vi "Text control 2 v3.6.vi"() -> ()   [LabVIEW 2016]
panel:
  in  "Delay before read (ms)":u32=1000
  out "I vs Vd":cluster{"Y data in":dbl[], "X data in":dbl[]}[](graph)
  in  "Auto Reset":bool
  in  "Reset":bool
  out "Id min vs time":cluster{"Y data in":dbl[], "X data in":dbl[]}[](graph)
  in  "Time Offset":dbl caption="Set Start Time (s)"
  out "Total lines":i32
  out "Line running":i32
  in  "byte count":u32=64
  in  "Serial End Mode for Reads":u16(ring)=2 items=["None", "LastBit", "TermChar"]
  in  "Timeout (ms)":u32=10000
  in  "Enable Termination\nChar (T)":bool=TRUE
  in  "Termination char\n(0xA = '\\n' = LF)\n(0xD = '\\r' = CR)":u8=13 format="%.0x"
  in  "flow control":u16(ring) items=["None"=0, "XON/XOFF"=1, "RTS/CTS"=2, "DTR/DSR"=4]
  in  "stop bits":u16(ring)=10 items=["1.0"=10, "1.5"=15, "2.0"=20]
  in  "parity":u16(ring) items=["None", "Odd", "Even", "Mark", "Space"]
  in  "data bits":u16=8 min=5 max=8 step=1
  in  "VISA resource name":refnum<visa-resource-name>="COM6"
  in  "baud rate":u32=9600
  out "Serial port output":string
  out "error out":errorcluster
  in  "Units":u16(ring) items=["Seconds", "Minutes", "Hours"]
  out "Elapsed Time":dbl caption="Elapsed Time (s)"
  out "Id max vs time":cluster{"Y data in":dbl[], "X data in":dbl[]}[](graph)
  out "Ig":dbl format="%.2e"
  out "Id":dbl format="%.2e"
  out "Is":dbl format="%.2e"
  out "I vs Vg":cluster{"Y data in":dbl[], "X data in":dbl[]}[](graph)
  in  "Panel Controls 2":T1={"Emergency Stop"=refnum, "TransGraph Max"=1e-05, "Text/Graph (text=false)"=TRUE, "TransGraph Min"=1e-11} {"TransGraph Min" format="%.2e"; "TransGraph Max" format="%.2e"}
  out "Command running:":string="#output s 0 0 0 -0.008 0.008 0.002"
  in  "Standby":T2
  in  "Full Reset":bool
  in  "SMU4":cluster{"on/off":bool, "Voltage":dbl} {"Voltage" min=-100.0 max=100.0 format="%.2f"}
  in  "Source/Drain Range":u8(slide)=6 max=11 scale=0.0..11.0
  in  "Source/Drain\nRange mode":u16(ring) items=["Auto", "Limited", "Fixed"]
  in  "Gate Range":u8(slide)=6 max=11 scale=0.0..11.0
  in  "Gate Range\nmode":u16(ring) items=["Auto", "Limited", "Fixed"]
  in  "Gate":T3={"Gate Start"=0.0, "Gate Stop"=2.0, "Gate Step (linear only)"=1.0, "Gate Compliance"=0.0001, "Gate PComp"=0.0, "Range mode"=0, "Range"=6} {"Range" max=11 scale=0.0..11.0; "Range mode" items=["Auto", "Limited", "Fixed"]; "Gate PComp" format="%^.2e"; "Gate Compliance" format="%^.2e"; "Gate Step (linear only)" format="%^.4e"; "Gate Stop" format="%^.4e"; "Gate Start" format="%^.4e"}
  in  "Drain 2":T4={"Drain Start"=0.0, "Drain Stop"=2.0, "Drain Compliance"=0.0001, "Drain Step"=1.0, "Drain PComp"=0.0, "Range mode"=0, "Range"=6} {"Range" max=11 scale=0.0..11.0; "Range mode" items=["Auto", "Limited", "Fixed"]; "Drain PComp" format="%^.2e"; "Drain Step" format="%^.4e"; "Drain Compliance" format="%^.2e"; "Drain Stop" format="%^.4e"; "Drain Start" format="%^.4e"}
  in  "Timings 2":T5={"integration time"=0, "Short/Long integration time"=0.00064, "hold time (sec)"=0.0, "delay time (sec)"=0.0, "Step Time (0 disables)"=0.0, "sweep method"=0, "Pulse period"=0.005, "Base voltage"=0.0, "Pulse width"=0.0005} {"Pulse width" min=0.0005 max=0.1 step=0.0001 format="%.4f"; "Base voltage" format="%^.4e"; "Pulse period" min=0.005 max=1.0 step=0.0001 format="%.4f"; "sweep method" items=["Continuous", "Pulsed"]; "Step Time (0 disables)" format="%.2f"; "delay time (sec)" format="%.4f"; "hold time (sec)" format="%.4f"; "Short/Long integration time" format="%^.0e"; "integration time" scale=0.0..2.0}
  in  "Panel Controls":T6={"Emergency Stop"=refnum, "TransGraph Max"=1e-05, "Text/Graph (text=false)"=TRUE} {"TransGraph Max" format="%.2e"}
  in  "Interrupt run":bool
  in  "Drain: Compliance":dbl=0.001 format="%.8f"
  in  "Gate: Compliance":dbl=0.001 format="%.8f"
  out "Path":path=path "C:/users/rlp38/09Apr2009LTtesting/test2.txt"
  in  "hold time /s":dbl format="%.2f"
  in  "delay time /s":dbl format="%.2f"
  in  "integration time":u32(slide) max=2 step=1 scale=0.0..2.0
  in  "Integration time (short)":dbl=0.0019 min=8e-05 max=0.0019 step=8e-05 format="%^.0e"
  in  "Integration time (long)":dbl=0.32 min=0.04 max=2.0 step=0.02 format="%.2f"
  in  "Step delay /s":dbl format="%.2f"
  in  "Program":string="#pulsedstressV d 0.03 20 0 0.5 0.0827 5\n#\n#itime s\n#gaterangemode l\n#drainrangemode l\n#serial /1Q\n#serial /1ZR\n#pulsed on 0.05 0 0.02\n#transfer d 1 -1 -0.1 -1 -1 0\n#wait-min 1\n#transfer d 1 -1 -0.1 -1 -1 0\n#output d 0 -1 -0.5 0 -1 -0.1\n#transfer d -10 40 1 5 40 35\n#transfer d -10 40 1 5 40 35\n#output d 0 40 20 0 40 1\n#\n#\n#sample 1 0.008 221 6 0.003\n#samplei 400e-6 200 6 0.002 0.1\n#vsu2pulse -10 4\n#\n#stressV 0.016 0.03 2e-4 0.1e-3 11\n#stressI 220e-7 0.08 15\n#transfer s -1 1 0.5 -0.005 0.005 0.005\n#output s 0 0 0 -0.008 0.008 0.002"
  # "Serial port settings"
  # "Time"
  # "Syntax:\nitime [s|m|l]\ngaterangemode [a|l|f]\ndrainrangemode [a|l|f]\npulsed [on|off] PulsePeriod(sec) PulseBaseVoltage PulseONWidth(sec)\nstandby [on l off]\nwait NumMilliseconds\nwait-min NumMinutes\n# texthere = comment\ntransfer [s|d] VgStart VgStop VgStep VdStart VdStop VdStep\noutput [s|d] VgStart VgStop VgStep VdStart VdStop VdStep\nsample Vg Vd NumSamples Time(s) SampleInterval(s)\nsamplei Idg NumSamples Time(s) SampleInterval(s) VDGcompliance\n100 samples is approximately 13 seconds with medium integration\n# if in doubt use SampleInterval(s) = 0.004\nstressV VG VD IGcompliance IDcompliance Duration(sec)\nstressI IDG VDGcompliance Duration(sec)\nvsu2pulse Bias Duration(s)\npulsedstressV [s|d] VEstop VgON VgOFF Period(s) PulseONwidth(s) Vd\nsample-fpp Vg Vd NumSamples Time\nresample-fpp Vg Vd\ntransfer-fpp [s|d] VgStart VgStop VgStep VdStart VdStop VdStep\noutput-fpp [s|d] VgStart VgStop VgStep VdStart VdStop VdStep\nserial SerialPortCommand\n\nSPM OEM Pump Syntax (x: pump number, use 1 if only one pump):\n/xQ: query\n/xZR: initialize pump\n/xIn: turn to port number n (clockwise)\n/xOn: turn to port number n (counterclockwise)"
  # "1\n2\n3\n4\n5\n6\n7\n8\n9\n10\n11\n12\n13\n14\n15\n16\n17\n18\n19\n20\n21\n22\n23\n24\n25"
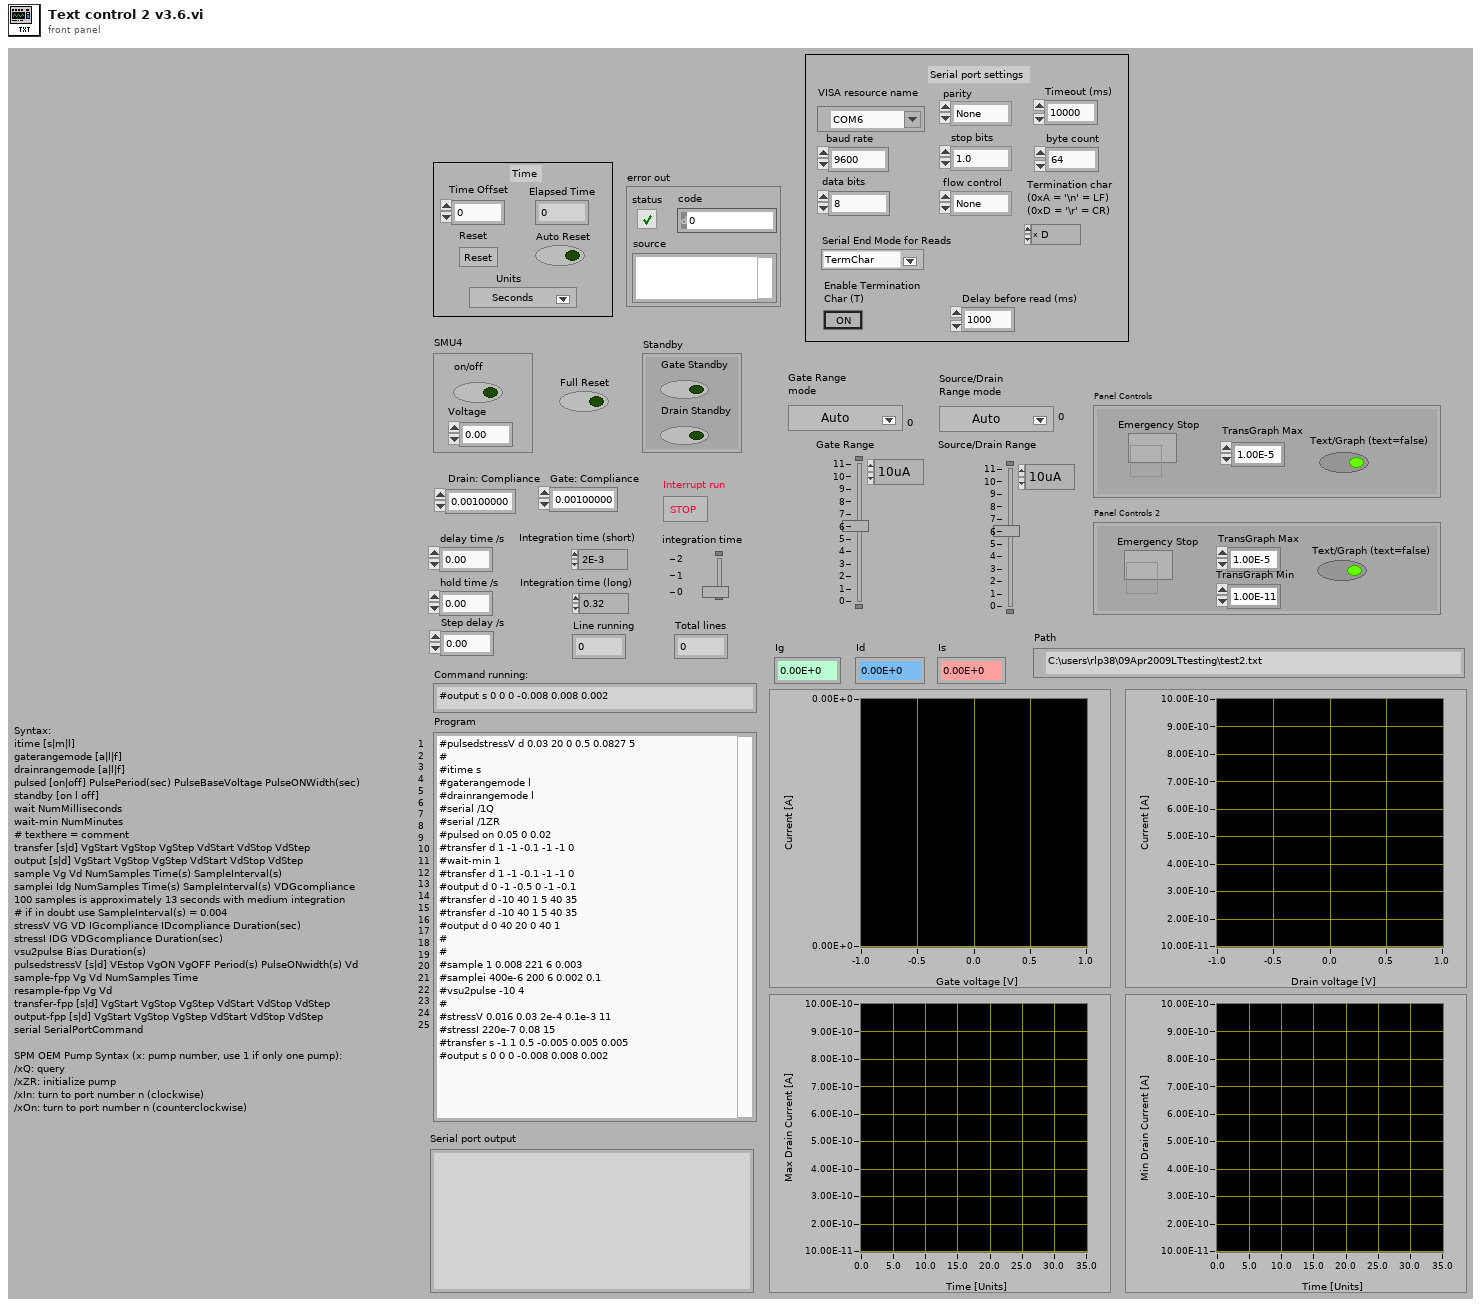
[diagram p1: front panel]
types:
  T1 = cluster{"Emergency Stop":refnum<vi>, "TransGraph Max":dbl, "Text/Graph (text=false)":bool, "TransGraph Min":dbl}
  T2 = cluster{"Gate Standby":bool, "Drain Standby":bool}
  T3 = cluster{"Gate Start":dbl, "Gate Stop":dbl, "Gate Step (linear only)":dbl, "Gate Compliance":dbl, "Gate PComp":dbl, "Range mode":u16, "Range":u8}
  T4 = cluster{"Drain Start":dbl, "Drain Stop":dbl, "Drain Compliance":dbl, "Drain Step":dbl, "Drain PComp":dbl, "Range mode":u16, "Range":u8}
  T5 = cluster{"integration time":u32, "Short/Long integration time":dbl, "hold time (sec)":dbl, "delay time (sec)":dbl, "Step Time (0 disables)":dbl, "sweep method":u16, "Pulse period":dbl, "Base voltage":dbl, "Pulse width":dbl}
  T6 = cluster{"Emergency Stop":refnum<vi>, "TransGraph Max":dbl, "Text/Graph (text=false)":bool}
  T7 = enum16{"open", "replace", "create", "open or create", "replace or create", "replace or create with confirmation"}
  T8 = cluster{"V2 Start":dbl, "V2 Step":dbl, "Number of points":i32}
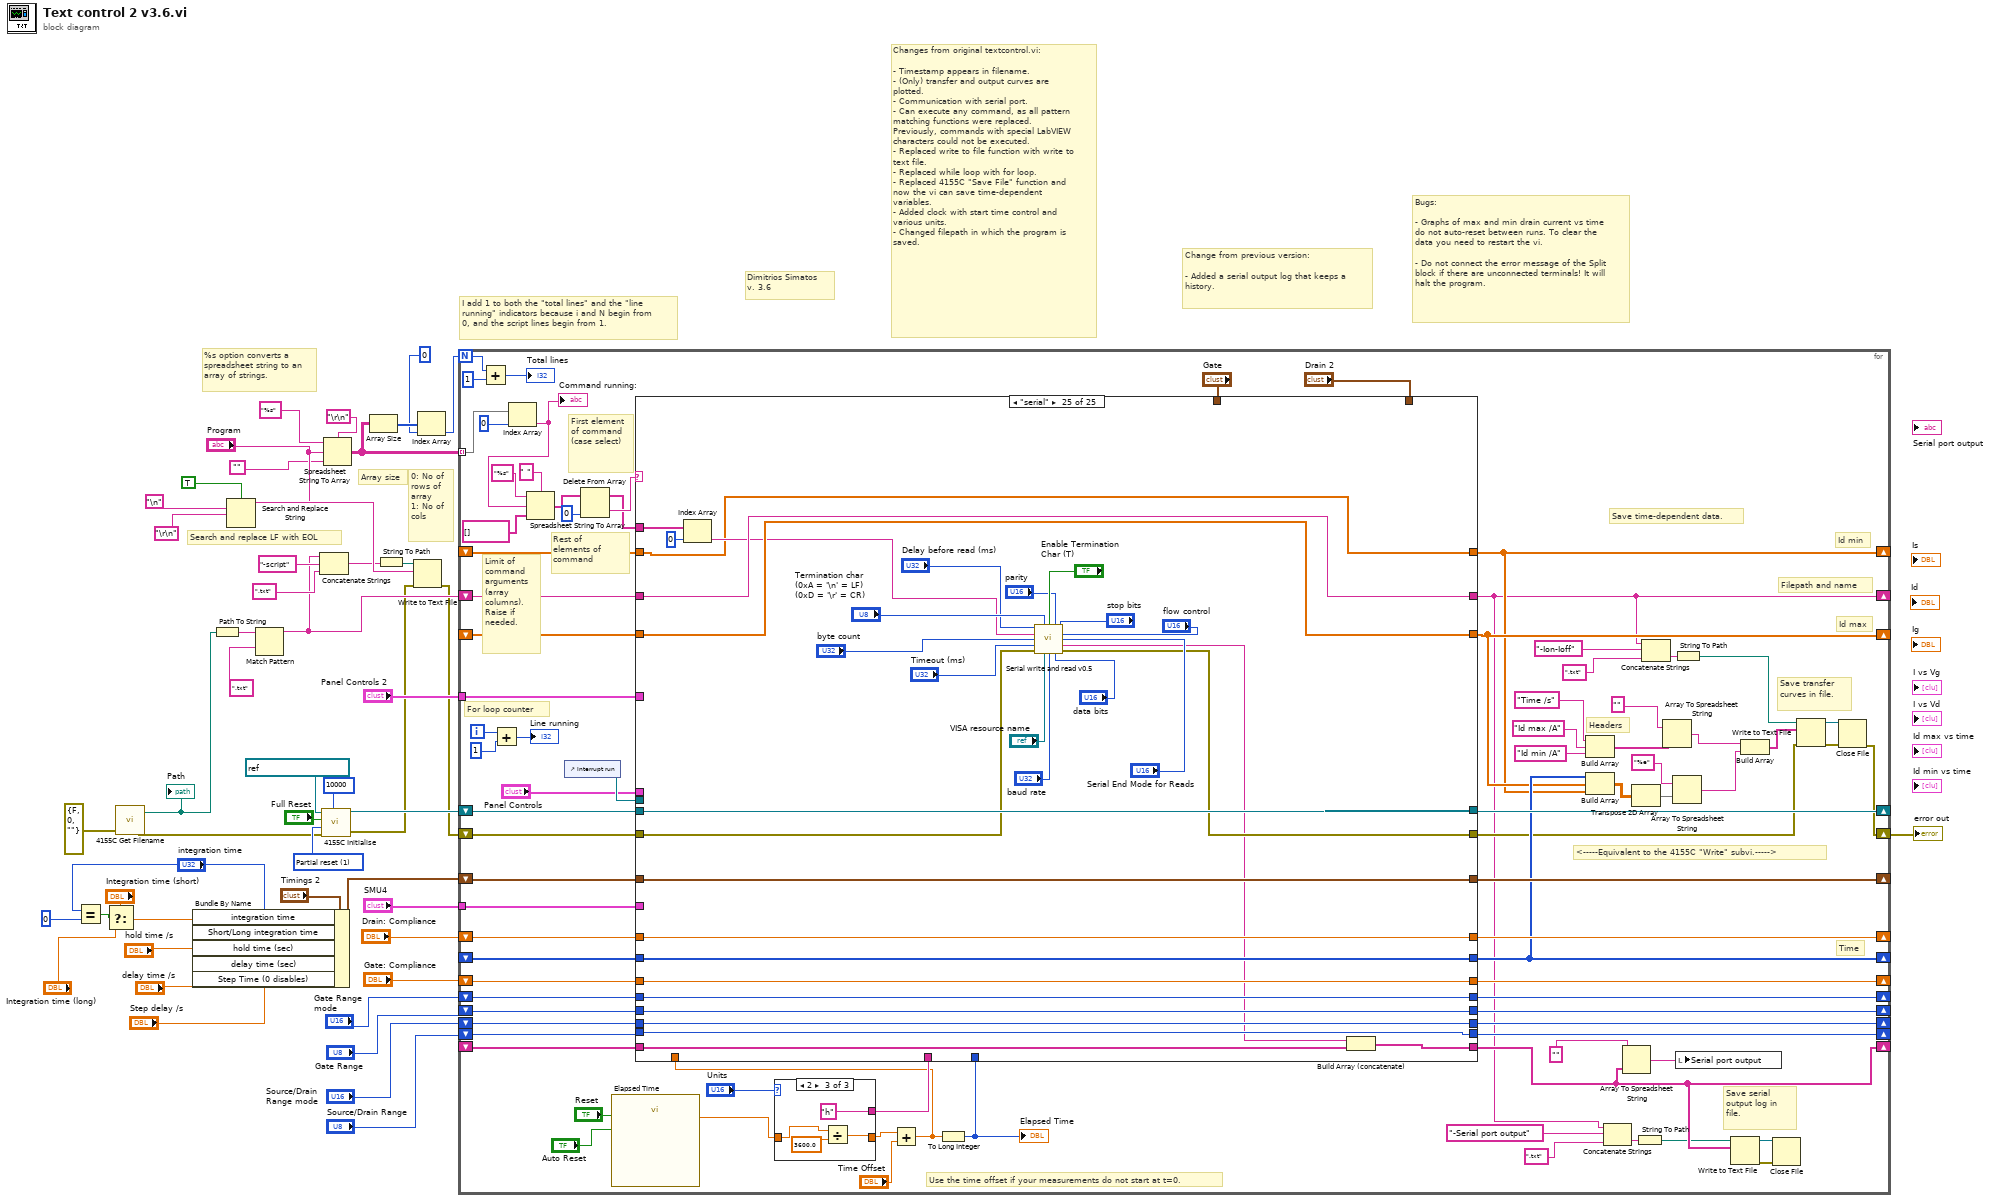
[diagram p0: block diagram]
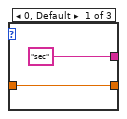
[diagram p2: hidden frame]
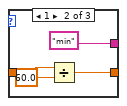
[diagram p3: hidden frame]
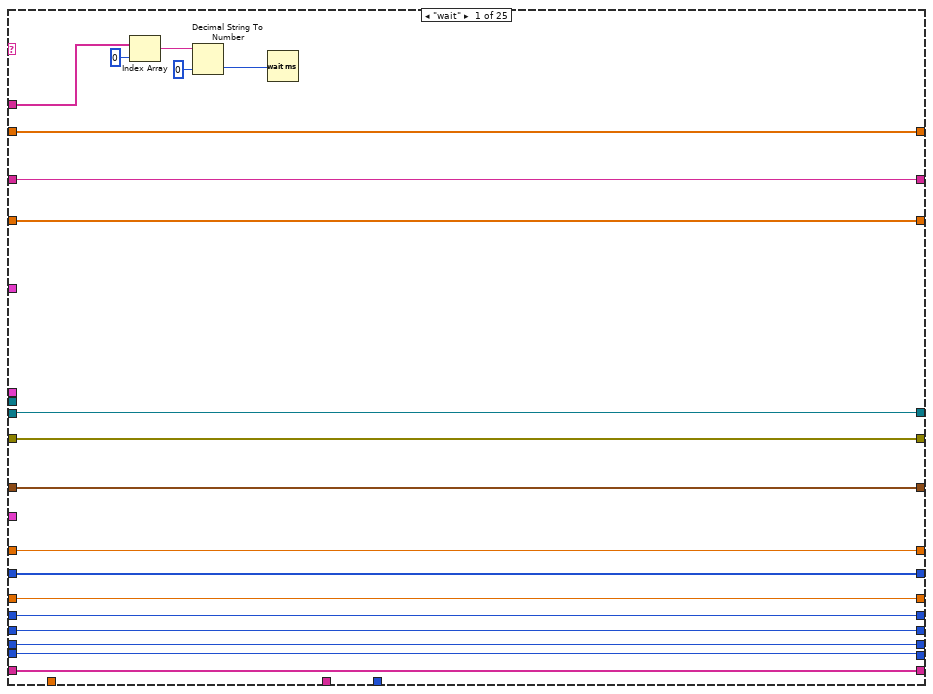
[diagram p4: hidden frame]
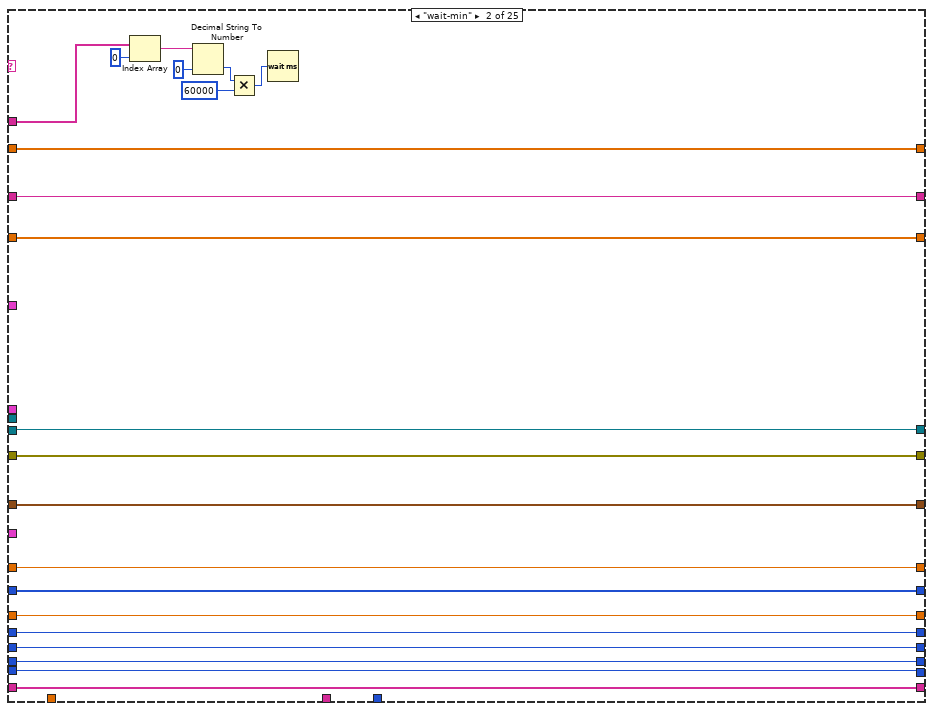
[diagram p5: hidden frame]
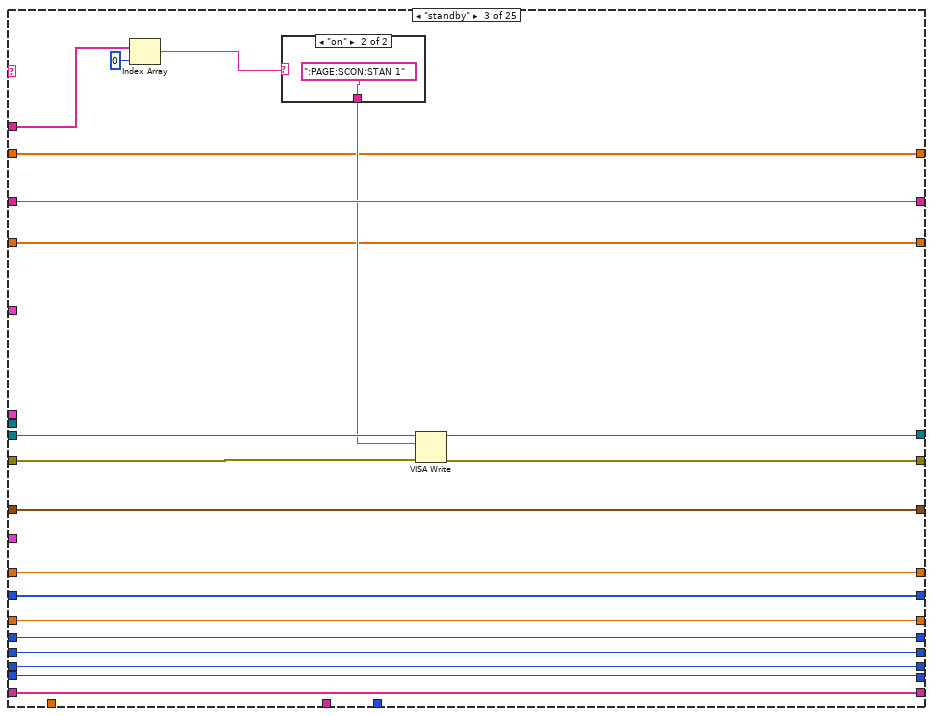
[diagram p6: hidden frame]
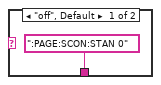
[diagram p7: hidden frame]
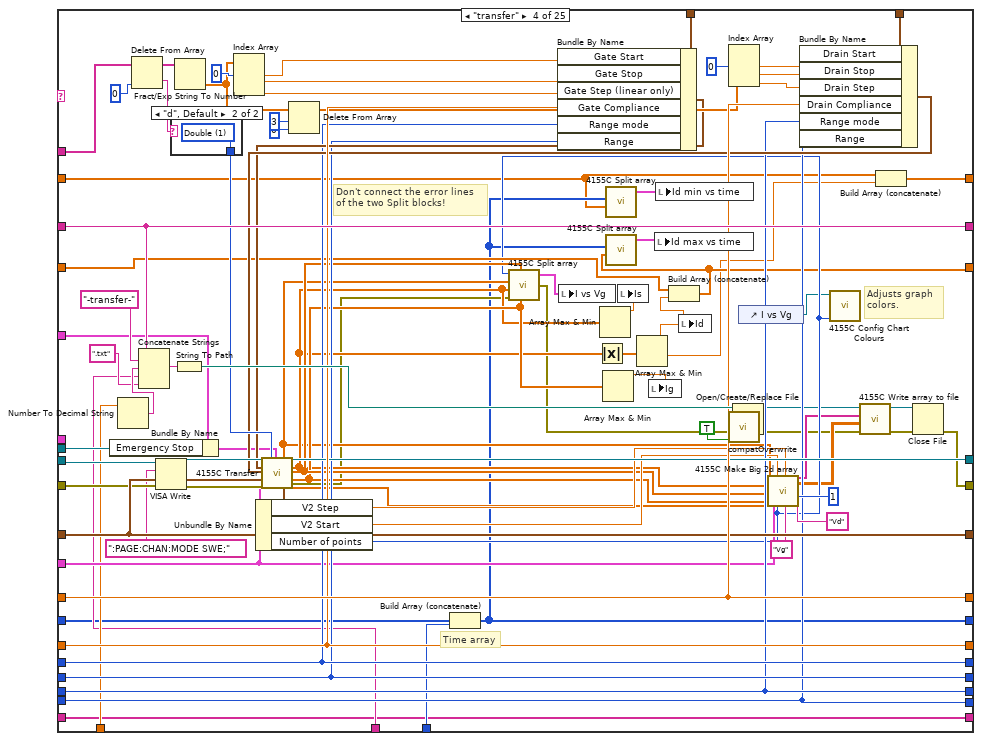
[diagram p8: hidden frame]
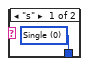
[diagram p9: hidden frame]
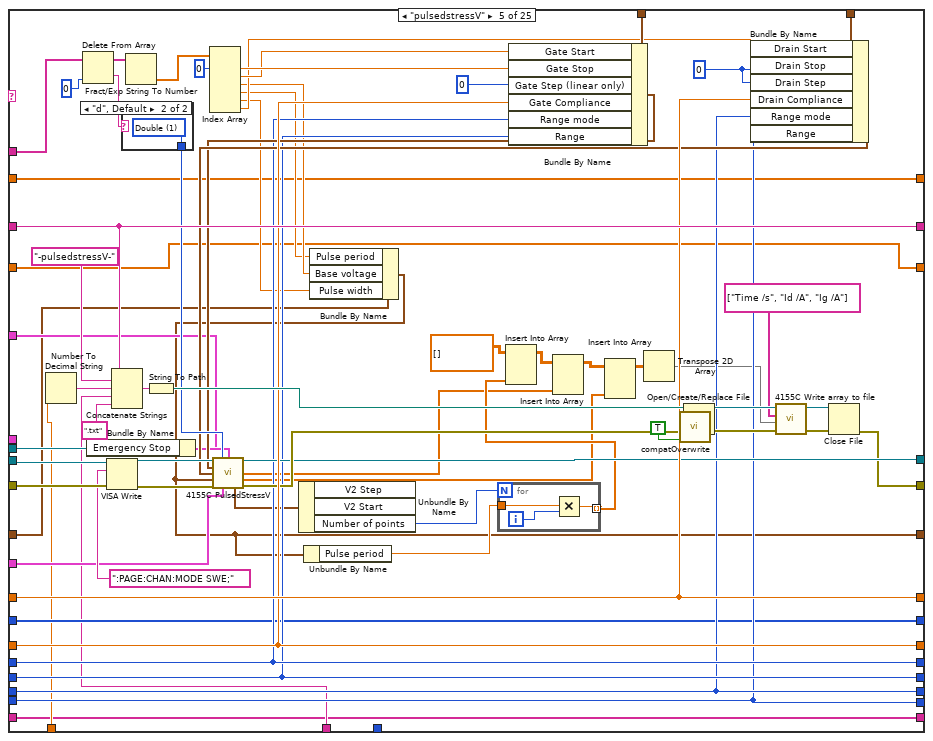
[diagram p10: hidden frame]
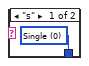
[diagram p11: hidden frame]
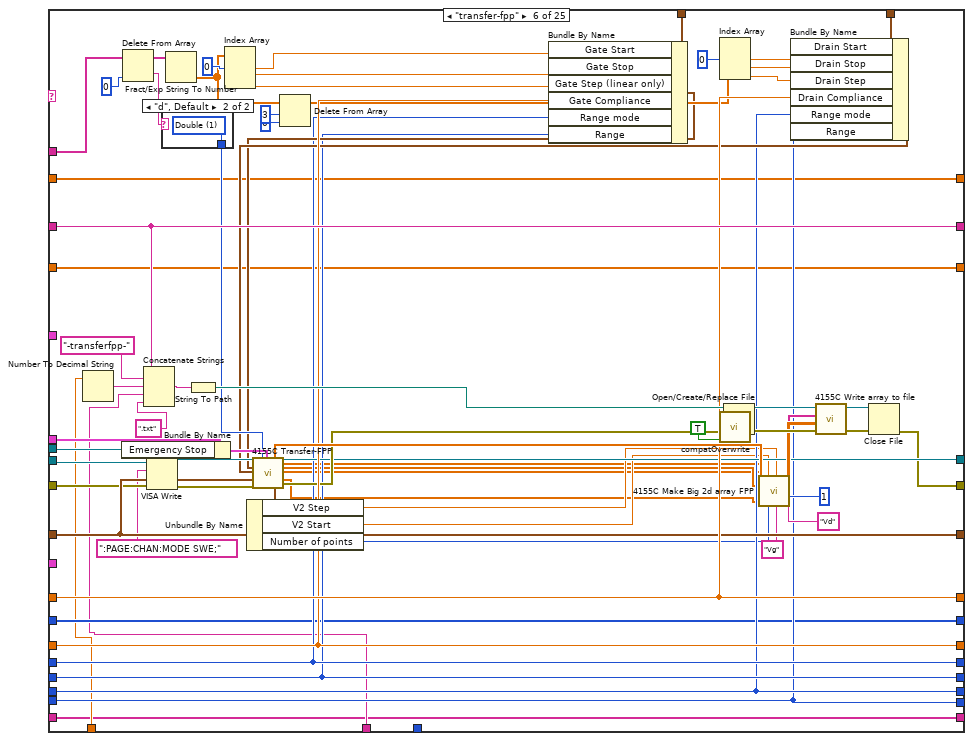
[diagram p12: hidden frame]
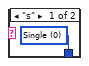
[diagram p13: hidden frame]
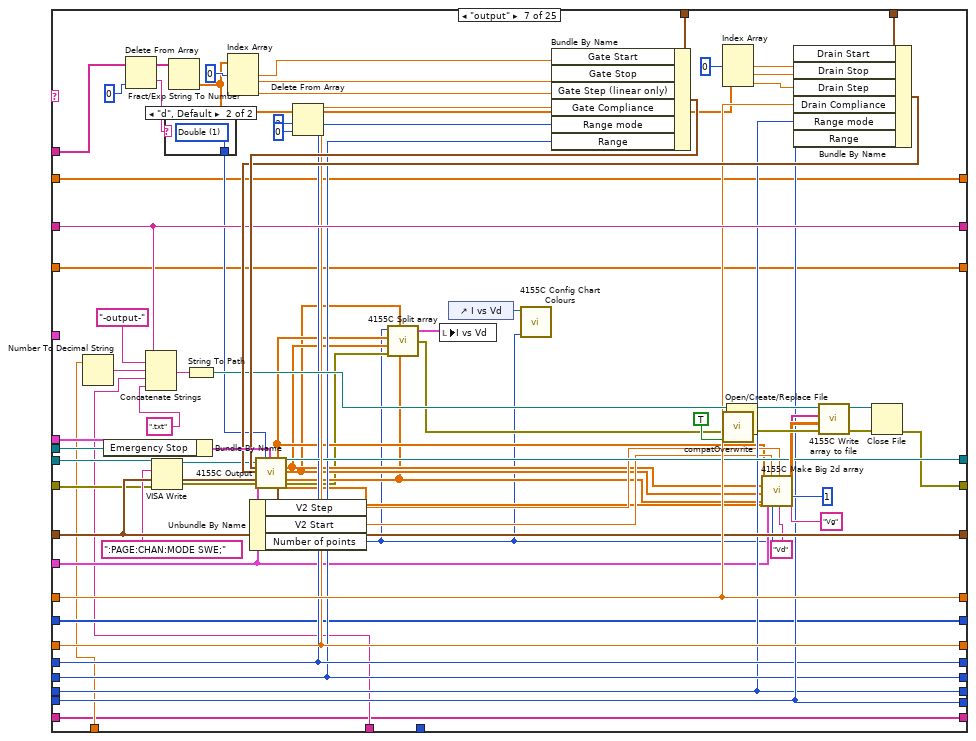
[diagram p14: hidden frame]
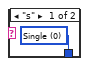
[diagram p15: hidden frame]
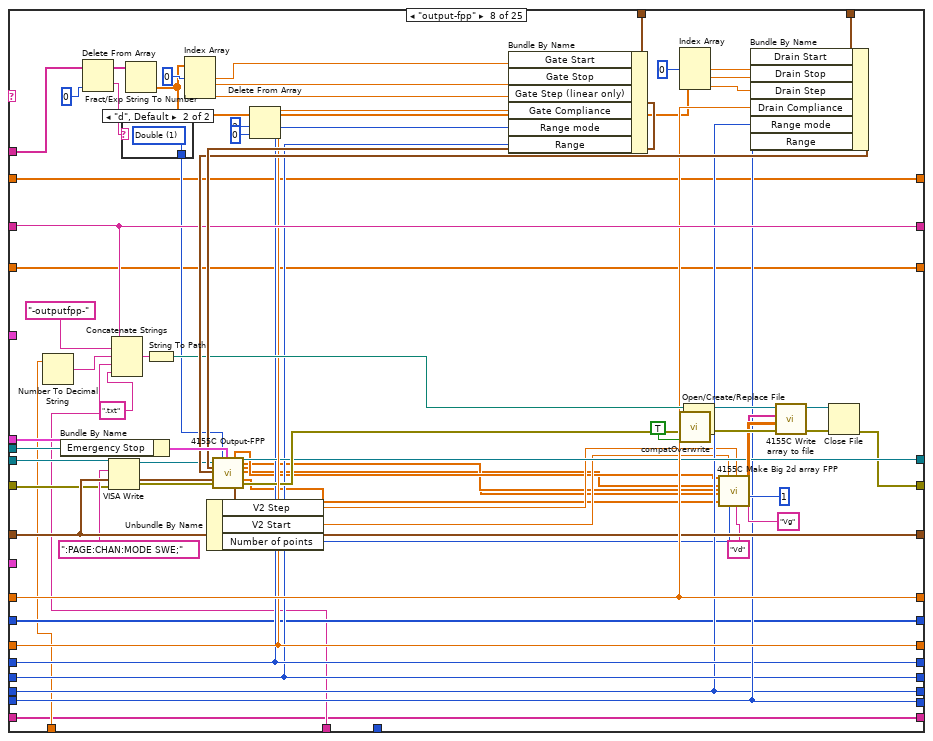
[diagram p16: hidden frame]
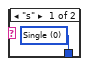
[diagram p17: hidden frame]
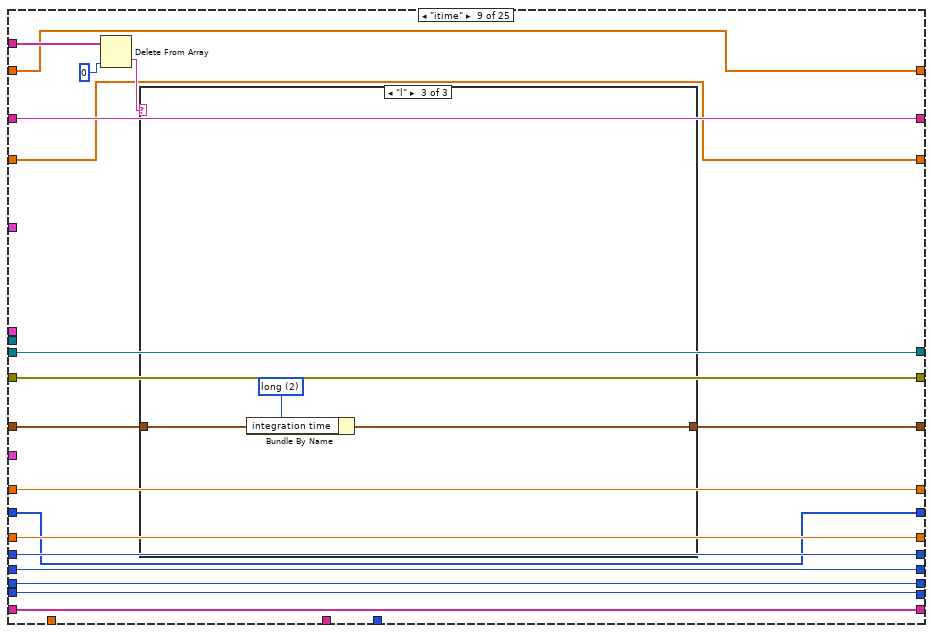
[diagram p18: hidden frame]
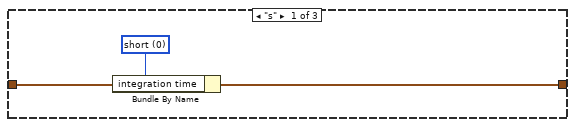
[diagram p19: hidden frame]
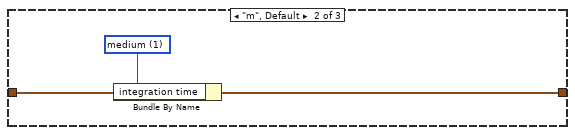
[diagram p20: hidden frame]
diagram:
  w40 = u16 1 items=["Reset All", "Partial reset"] ("Type of reset")
  # "I add 1 to both the \"total lines\" and the \"line running\" indicators because i and N begin from 0, and the script lines begin from 1."
  # "Bugs:\n\n- Graphs of max and min drain current vs time do not auto-reset between runs. To clear the data you need to restart the vi.\n\n- Do not connect the error message of the Split block if there are unconnected terminals! It will halt the program."
  # "Array size"
  # "%s option converts a spreadsheet string to an array of strings."
  # "0: No of rows of array\n1: No of cols"
  # "Change from previous version:\n\n- Added a serial output log that keeps a history."
  # "Dimitrios Simatos\nv. 3.6"
  # "Changes from original textcontrol.vi:\n\n- Timestamp appears in filename.\n- (Only) transfer and output curves are plotted.\n- Communication with serial port.\n- Can execute any command, as all pattern matching functions were replaced. Previously, commands with special LabVIEW characters could not be executed.\n- Replaced write to file function with write to text file.\n- Replaced while loop with for loop.\n- Replaced 4155C \"Save File\" function and now the vi can save time-dependent variables.\n- Added clock with start time control and various units.\n- Changed filepath in which the program is saved."
  # "Search and replace LF with EOL"
  n1 = Equal?(x="integration time", y=u32 0) -> (x = y?=w44:bool)
  n2 = Select(t="Integration time (short)", s=w44, f="Integration time (long)") -> (s? t:f=w48:dbl)
  n3 = call "4155C Get Filename.vi"("error in (no error)"=errorcluster {"status"=FALSE, "code"=0, "source"=""}) -> ("error out"=w35:errorcluster, "path"=w10:path)  [unwired: 2 in, 1 out]
  "Path" <- w10
  n4 = Bundle By Name(cluster="Timings 2", "integration time"="integration time", "Short/Long integration time"=w48, "hold time (sec)"="hold time /s", "delay time (sec)"="delay time /s", "Step Time (0 disables)"="Step delay /s") -> (w33:T5)
  n5 = Path To String(path=w10) -> (string=w11:string)
  n6 = Search and Replace String(replace all?=TRUE ("replace all? (F)"), input string="Program", search string="\n", replace string="\r\n") -> (result string=w23:string)  [unwired: 4 in, 3 out]
  n7 = Match Pattern(string=w11, regular expression=".txt") -> (before substring=w5:string)  [unwired: 1 in, 3 out]
  n8 = Concatenate Strings(w5, "-script" ("Prefix"), ".txt" ("regular expression")) -> (w4:string)
  n9 = call "4155C Initialise.vi"("VISA resource name in"=refnum<visa-resource-name> "GPIB0::14::INSTR", "Reset"="Full Reset", "Type of reset"=w40, "error in (no error)"=w35, "VISA Timeout Value"=u32 10000) -> ("VISA Resource Name out"=w34:refnum<visa-resource-name>, "error out"=w2:errorcluster)
  n10 = Spreadsheet String To Array(delimiter (Tab)="\r\n", format string="%s", spreadsheet string="Program", array type (2D Dbl)="") -> (array=w14:string[][])
  n11 = Array Size(array=w14) -> (size(s)=w18:i32[])
  n12 = String To Path(string=w4) -> (path=w3:path)
  n13 = Write to Text File(file (use dialog)=w3, text=w23, error in=w2) -> (error out=w1:errorcluster)  [unwired: 1 in, 2 out]
  n14 = Index Array(array=w18, index=0) -> (element=w16:i32)
  n15 = for {
    N: w16 -> [w66]
    tunnel: "SMU4" -> [w112]
    shift-left: "Source/Drain Range" -> [w117]
    shift-right: [w113] -> _
    shift-left: "Source/Drain\nRange mode" -> [w118]
    shift-right: [w114] -> _
    shift-left: "Gate Range" -> [w119]
    shift-right: [w115] -> _
    shift-left: "Gate Range\nmode" -> [w120]
    shift-right: [w116] -> _
    shift-left: "Gate: Compliance" -> [w129]
    shift-right: [w125] -> _
    shift-left: "Drain: Compliance" -> [w130]
    shift-right: [w126] -> _
    shift-left: w33 -> [w131]
    shift-right: [w127] -> _
    shift-left: w1 -> [w132]
    shift-right: [w74] -> w9
    shift-left: w34 -> [w133]
    shift-right: [w128] -> _
    shift-left: w5 -> [w134]
    shift-right: [w50] -> _
    tunnel: "Panel Controls 2" -> [w111]
    shift-right: [w79] -> _
    shift-left: _ -> [w110]
    shift-right: [w80] -> _
    shift-left: _ -> [w106]
    tunnel: w14 -> [w104] mode=indexing
    shift-right: [w72] -> _
    shift-left: _ -> [w73]
    shift-right: [w55] -> _
    shift-left: _ -> [w58]
    i -> [w61]
    # "Save serial output log in file."
    # "For loop counter"
    # "<-----Equivalent to the 4155C \"Write\" subvi.----->"
    # "Headers"
    # "Save transfer curves in file."
    # "Filepath and name"
    # "Save time-dependent data."
    # "Use the time offset if your measurements do not start at t=0."
    # "Time"
    # "Rest of elements of command"
    # "Id min"
    # "Id max"
    # "Limit of command arguments (array columns). Raise if needed."
    # "First element of command\n(case select)"
    n16 = Add(x=w66, y=1) -> (x+y=→"Total lines":i32)
    n17 = Add(x=w61, y=1) -> (x+y=→"Line running":i32)
    n18 = Index Array(array=w104, index=0 ("line index")) -> (element=w99:string)
    "Command running:" <- w99
    n19 = Spreadsheet String To Array(delimiter (Tab)=" ", format string="%s", spreadsheet string=w99, array type (2D Dbl)=string[] []) -> (array=w96:string[])
    n20 = control-ref of="Interrupt run"() -> (w124:refnum<vi>)
    n21 = Delete From Array(array=w96, index=0) -> (deleted portion=w97:string, array with subset deleted=w95:string[])  [unwired: 1 in]
    n22 = call "Elapsed Time"("Reset"="Reset", "Auto Reset"="Auto Reset") -> ("Elapsed Time (s)"=w107:dbl)  [unwired: 10 in, 7 out]
    n23 = case shown="2" "Units" {
      tunnel: ["sec" "min" "h"] -> w108
      tunnel: [w135 w139 w142] -> w68
      tunnel: w107 -> [w135 w138 w143]
      frame 0, Default {
      }
      frame 1 {
        n24 = Divide(x=w138, y=60.0) -> (x/y=w139:dbl)
      }
      frame 2 {
        n25 = Divide(x=w143, y=3600.0) -> (x/y=w142:dbl)
      }
    }
    n26 = Add(x=w68, y="Time Offset") -> (x+y=w67:dbl)
    n27 = To Long Integer(number=w67) -> (32bit integer=w105:i32)
    "Elapsed Time" <- w105
    n28 = case shown="\"serial\"" w97 {
      tunnel: w95 -> [w163 w184 w204 w281 w347 w418 w495 w567 w607 w635 w664 w691 w714 w730 _ _ w840 w903 _ w972 w1018 w1062 w1134 w1198 w1210]
      tunnel: w134 -> [w158 w180 w202 w288 w354 w426 w502 w575 w596 w624 w656 w684 w708 w723 w744 w788 w818 w885 w918 w959 w1005 w1050 w1128 w1194 w1212]
      tunnel: w133 -> [w157 w179 w193 w259 w338 w395 w471 w543 w597 w625 w657 w685 w709 w724 w749 w790 w846 w909 w922 w978 w1024 w1068 w1140 w1152 w1216]
      tunnel: w132 -> [w156 w178 w192 w258 w337 w394 w468 w540 w598 w626 w658 w686 w710 w725 w748 w761 w845 w908 w921 w977 w1023 w1067 w1139 w1151 w1215]
      tunnel: w131 -> [w155 w177 w201 w284 w313 w422 w498 w571 w606 w634 w655 w683 w707 w722 w747 w785 w809 w877 w927 w952 w998 w1043 w1127 w1193 w1217]
      tunnel: w130 -> [w154 w176 w200 w286 w352 w424 w500 w573 w605 w633 w663 w690 w713 w729 w746 w770 w844 w907 w930 w976 w1022 w1066 w1138 w1202 w1218]
      tunnel: w129 -> [w153 w175 w199 w285 w351 w423 w499 w572 w604 w632 w662 w689 w712 w728 w745 w771 w819 w886 w929 w960 w1006 w1051 w1129 w1195 w1220]
      tunnel: [w157 w179 w191 w283 w349 w420 w497 w569 w597 w625 w657 w685 w709 w724 w749 w790 w810 w859 w920 w953 w999 w1044 w1080 w1154 w1216] -> w128
      tunnel: [w156 w178 w190 w282 w348 w419 w496 w568 w598 w626 w658 w686 w710 w725 w748 w760 w820 w860 w919 w961 w1007 w1052 w1079 w1153 w1214] -> w75
      tunnel: [w155 w177 w201 w284 w309 w422 w498 w571 w599 w627 w655 w683 w707 w722 w747 w785 w809 w877 w927 w952 w998 w1043 w1127 w1193 w1217] -> w127
      tunnel: [w154 w176 w200 w286 w352 w424 w500 w573 w605 w633 w663 w690 w713 w729 w746 w770 w844 w907 w930 w976 w1022 w1066 w1138 w1202 w1218] -> w126
      tunnel: [w153 w175 w199 w285 w351 w423 w499 w572 w604 w632 w662 w689 w712 w728 w745 w771 w819 w886 w929 w960 w1006 w1051 w1129 w1195 w1220] -> w125
      tunnel: [w158 w180 w202 w288 w354 w426 w502 w575 w596 w624 w656 w684 w708 w723 w744 w788 w818 w885 w918 w959 w1005 w1050 w1128 w1194 w1212] -> w50
      tunnel: w124 -> [_ _ _ w291 w358 w431 w506 w579 _ _ _ _ _ _ _ _ w815 w882 _ w958 w1004 w1049 w1100 w1170 _]
      tunnel: "Gate" -> [_ _ _ w268 w341 w405 w482 w554 _ _ _ _ _ _ _ _ _ _ _ _ _ _ _ _ _]
      tunnel: "Drain 2" -> [_ _ _ w267 w340 w404 w481 w553 _ _ _ _ _ _ _ _ _ _ _ _ _ _ _ _ _]
      tunnel: "Panel Controls" -> [_ _ _ _ _ w403 w480 w552 _ _ _ _ _ _ _ _ _ _ _ _ _ _ _ _ _]
      tunnel: w120 -> [w152 w174 w198 w252 w331 w388 w466 w538 w603 w631 _ w682 w706 w721 w743 w772 w805 w873 w923 w948 w994 w1039 w1123 w1189 w1221]
      tunnel: w119 -> [w151 w173 w197 w251 w330 w387 w465 w537 w602 w630 w661 _ w697 w727 w742 w773 w806 w874 w924 w949 w995 w1040 w1124 w1190 w1222]
      tunnel: w118 -> [w150 w172 w196 w250 w329 w386 w464 w536 w601 w629 w660 w688 w711 _ w741 w774 w807 w875 w925 w950 w996 w1041 w1125 w1191 w1223]
      tunnel: w117 -> [w149 w171 w195 w249 w328 w385 w467 w539 w600 w628 w659 w687 _ w726 w740 w775 w808 w876 w926 w951 w997 w1042 w1126 w1192 w1224]
      tunnel: [w152 w174 w198 w252 w331 w388 w466 w538 w603 w631 w654 w682 w706 w721 w743 w772 w805 w873 w923 w948 w994 w1039 w1123 w1189 w1221] -> w116
      tunnel: [w151 w173 w197 w251 w330 w387 w465 w537 w602 w630 w661 w674 w697 w727 w742 w773 w806 w874 w924 w949 w995 w1040 w1124 w1190 w1222] -> w115
      tunnel: [w150 w172 w196 w250 w329 w386 w464 w536 w601 w629 w660 w688 w711 w720 w741 w774 w807 w875 w925 w950 w996 w1041 w1125 w1191 w1223] -> w114
      tunnel: [w149 w171 w195 w249 w328 w385 w467 w539 w600 w628 w659 w687 w698 w726 w740 w775 w808 w876 w926 w951 w997 w1042 w1126 w1192 w1224] -> w113
      tunnel: w112 -> [_ _ _ w244 w325 _ w460 _ _ _ _ _ _ _ _ _ _ _ _ _ _ _ _ _ _]
      tunnel: w111 -> [_ _ _ w242 w324 _ _ _ _ _ _ _ _ _ _ _ _ _ _ _ _ _ _ _ _]
      tunnel: [w148 w167 w188 w219 w301 w375 w457 w525 w595 w622 w653 w673 w696 w719 w739 w756 w797 w857 w917 w937 w987 w1033 w1077 w1147 w1213] -> w79
      tunnel: w110 -> [w148 w167 w188 w233 w301 w375 w457 w525 w595 w622 w653 w673 w696 w719 w739 w756 w797 w857 w917 w937 w987 w1033 w1077 w1147 w1213]
      tunnel: w67 -> [_ _ _ w229 w298 w373 w454 w522 _ _ _ _ _ _ _ w754 w795 w854 _ w934 w984 w1030 w1074 w1143 _]
      tunnel: w108 -> [_ _ _ w226 w297 w371 w453 w521 _ _ _ _ _ _ _ w752 w793 w853 _ w933 w983 w1029 w1073 w1144 _]
      tunnel: w105 -> [_ _ _ w220 _ _ _ _ _ _ _ _ _ _ _ _ _ _ _ _ _ _ _ _ _]
      tunnel: [w147 w166 w187 w217 w300 w374 w456 w524 w594 w621 w652 w672 w695 w718 w738 w755 w796 w856 w916 w936 w986 w1032 w1076 w1146 w1219] -> w80
      tunnel: w106 -> [w147 w166 w187 w225 w300 w374 w456 w524 w594 w621 w652 w672 w695 w718 w738 w755 w796 w856 w916 w936 w986 w1032 w1076 w1146 w1219]
      tunnel: [w146 w165 w186 w215 w296 w370 w452 w520 w593 w620 w651 w671 w694 w717 w737 w751 w792 w852 w915 w932 w982 w1028 w1072 w1142 w1207] -> w72
      tunnel: w73 -> [w146 w165 w186 w214 w296 w370 w452 w520 w593 w620 w651 w671 w694 w717 w737 w751 w792 w852 w915 w932 w982 w1028 w1072 w1142 w1207]
      tunnel: [w145 w164 w185 w207 w295 w369 w442 w519 w592 w619 w650 w670 w693 w716 w736 w750 w791 w851 w914 w931 w981 w1027 w1071 w1141 w1205] -> w55
      tunnel: w58 -> [w145 w164 w185 w207 w295 w369 w442 w519 w592 w619 w650 w670 w693 w716 w736 w750 w791 w851 w914 w931 w981 w1027 w1071 w1141 w1204]
      frame "wait" {
        n29 = Index Array(array=w163, index=0 ("Index")) -> (element=w161:string)
        n30 = Decimal String To Number(string=w161, default (0L)=u32 0) -> (number=w160:u32)  [unwired: 1 in, 1 out]
        n31 = Wait (ms)(milliseconds to wait=w160) -> ()  [unwired: 1 out]
      }
      frame "wait-min" {
        n32 = Index Array(array=w184, index=0 ("Index")) -> (element=w182:string)
        n33 = Decimal String To Number(string=w182, default (0L)=u32 0) -> (number=w170:u32)  [unwired: 1 in, 1 out]
        n34 = Multiply(x=w170, y=u32 60000) -> (x*y=w169:u32)
        n35 = Wait (ms)(milliseconds to wait=w169) -> ()  [unwired: 1 out]
      }
      frame "standby" {
        n36 = Index Array(array=w204, index=0 ("Index")) -> (element=w194:string)
        n37 = case shown="\"on\"" w194 {
          tunnel: [":PAGE:SCON:STAN 0" ":PAGE:SCON:STAN 1"] -> w189
          frame "off", Default {
          }
          frame "on" {
          }
        }
        n38 = VISA Write(VISA resource name=w193, write buffer=w189, error in (no error)=w192) -> (VISA resource name out=w191:refnum<visa-resource-name>, error out=w190:errorcluster)  [unwired: 1 out]
      }
      frame "transfer" {
        # "Don't connect the error lines\nof the two Split blocks!"
        # "Adjusts graph colors."
        # "Time array"
        n39 = Bundle By Name(cluster=w242, "Emergency Stop"=w291) -> (w243:T1)
        n40 = Number To Decimal String(number=w229) -> (decimal integer string=w228:string)  [unwired: 1 in]
        n41 = Delete From Array(array=w281, index=0 ("Index")) -> (deleted portion=w279:string, array with subset deleted=w278:string[])  [unwired: 1 in]
        n42 = Concatenate Strings(w288, "-transfer-" ("Prefix"), w228, w226, ".txt" ("Suffix")) -> (w290:string)
        n43 = VISA Write(VISA resource name=w259, write buffer=":PAGE:CHAN:MODE SWE;" ("write buffer (\"\")"), error in (no error)=w258) -> (VISA resource name out=w256:refnum<visa-resource-name>, error out=w257:errorcluster)  [unwired: 1 out]
        n44 = case shown="\"d\", Default" w279 {
          tunnel: [w293 w294] -> w277
          frame "s" {
            w293 = u16 0 items=["Single", "Double"] ("sweep mode")
          }
          frame "d", Default {
            w294 = u16 1 items=["Single", "Double"] ("sweep mode")
          }
        }
        n45 = String To Path(string=w290) -> (path=w287:path)
        n46 = Fract/Exp String To Number(string=w278) -> (number=w263:dbl[])  [unwired: 3 in, 1 out]
        n47 = Index Array(array=w263, index #1=0 ("Index")) -> (element #1=w276:dbl, element #2=w275:dbl, element #3=w274:dbl)  [unwired: 2 in]
        n48 = Delete From Array(array=w263, length=3 ("Length"), index=0 ("Index")) -> (array with subset deleted=w261:dbl[])  [unwired: 1 out]
        n49 = Build Array (concatenate)(w225, w220) -> (w217:i32[])
        n50 = Bundle By Name(cluster=w268, "Gate Start"=w276, "Gate Stop"=w275, "Gate Step (linear only)"=w274, "Gate Compliance"=w285, "Range mode"=w252, "Range"=w251) -> (w253:T3)
        n51 = call "4155C Split array.vi"("X data in"=w217, "Y1 data in"=w214) -> ("Array of clusters"=w218:cluster{"Y data in":dbl[], "X data in":dbl[]}[])  [unwired: 5 in, 1 out]
        n52 = local write "Id min vs time"(w218) -> ()
        n53 = Index Array(array=w261, index #1=0 ("Index")) -> (element #1=w271:dbl, element #2=w270:dbl, element #3=w269:dbl)  [unwired: 2 in]
        n54 = call <vilib>:"compatOverwrite.vi"("overwrite (F)"=TRUE) -> ("overwrite?"=w241:T7)
        n55 = control-ref of="I vs Vg"() -> (w230:refnum<vi>)
        n56 = Bundle By Name(cluster=w267, "Drain Start"=w271, "Drain Stop"=w270, "Drain Step"=w269, "Drain Compliance"=w286, "Range mode"=w250, "Range"=w249) -> (w254:T4)
        n57 = call "4155C Transfer.vi"("VISA resource name in"=w256, "Gate"=w253, "Drain"=w254, "Timings"=w284, "error in (no error)"=w257, "SMU4"=w244, "sweep mode"=w277, "Panel Controls"=w243) -> ("VG"=w234:dbl[], "Outparams"=w248:T8, "VISA Resource Name out"=w283:refnum<visa-resource-name>, "IS"=w235:dbl[], "ID"=w240:dbl[], "IG"=w236:dbl[], "error out"=w221:errorcluster, "SMU4"=w245:dbl[])  [unwired: 12 in]
        n58 = Unbundle By Name(w248) -> ("V2 Step"=w247:dbl, "V2 Start"=w246:dbl, "Number of points"=w231:i32)
        n59 = call "4155C Split array.vi"("Number of VAR2 steps"=w231, "Y2 data in"=w240, "X data in"=w234, "Y1 data in"=w235, "Y3 data in"=w236, "error in (no error)"=w221) -> ("Array of clusters"=w224:cluster{"Y data in":dbl[], "X data in":dbl[]}[], "error out"=w222:errorcluster)  [unwired: 1 in]
        n60 = local write "I vs Vg"(w224) -> ()
        n61 = Absolute Value(x=w235) -> (abs(x)=w239:dbl[])
        n62 = Array Max & Min(array=w235) -> (max value=w237:dbl)  [unwired: 3 out]
        n63 = Array Max & Min(array=w236) -> (max value=w238:dbl)  [unwired: 3 out]
        n64 = local write "Is"(w237) -> ()
        n65 = Array Max & Min(array=w239) -> (max value=w232:dbl, min value=w216:dbl)  [unwired: 2 out]
        n66 = local write "Ig"(w238) -> ()
        n67 = Build Array (concatenate)(w233, w232) -> (w219:dbl[])
        n68 = call "4155C Split array.vi"("X data in"=w217, "Y1 data in"=w219) -> ("Array of clusters"=w223:cluster{"Y data in":dbl[], "X data in":dbl[]}[])  [unwired: 5 in, 1 out]
        n69 = local write "Id max vs time"(w223) -> ()
        n70 = local write "Id"(w232) -> ()
        n71 = Open/Create/Replace File(file path (use dialog)=w287, error in=w222, operation (0:open)=w241) -> (refnum out=w212:refnum<file>, error out=w210:errorcluster)  [unwired: 3 in, 1 out]
        n72 = call "4155C Make Big 2d array.vi"("1D Var1"=w234, "1d IS"=w235, "1d ID"=w240, "1d IG"=w236, "1d SMU4"=w245, "SMU4"=w244, "VAR2 START"=w246, "Number of VAR2 steps"=w231, "VAR2 STEP"=w247, "VAR1 Name"="Vg", "Decimal places in header"=i8 1, "VAR2 Name"="Vd") -> ("Header array"=w213:string[], "Data array"=w211:dbl[][])  [unwired: 14 in]
        n73 = call "4155C Config Chart Colours.vi"("Numeric"=w231, "XY Graph 2"=w230) -> ()  [unwired: 6 in]
        n74 = call "4155C Write array to file.vi"("Byte Stream File Refnum"=w212, "Header"=w213, "Data Array"=w211, "error in (no error)"=w210) -> ("dup refnum"=w209:refnum<file>, "error out"=w208:errorcluster)  [unwired: 1 in]
        n75 = Build Array (concatenate)(w214, w216) -> (w215:dbl[])
        n76 = Close File(refnum=w209, error in=w208) -> (error out=w282:errorcluster)  [unwired: 1 out]
      }
      frame "pulsedstressV" {
        w307 = 0
        n77 = Number To Decimal String(number=w298) -> (decimal integer string=w355:string)  [unwired: 1 in]
        n78 = Delete From Array(array=w347, index=0 ("Index")) -> (deleted portion=w345:string, array with subset deleted=w344:string[])  [unwired: 1 in]
        n79 = Bundle By Name(cluster=w324, "Emergency Stop"=w358) -> (w326:T1)
        n80 = VISA Write(VISA resource name=w338, write buffer=":PAGE:CHAN:MODE SWE;" ("write buffer (\"\")"), error in (no error)=w337) -> (VISA resource name out=w335:refnum<visa-resource-name>, error out=w336:errorcluster)  [unwired: 1 out]
        n81 = Concatenate Strings(w354, "-pulsedstressV-" ("Substring"), w355, w297, ".txt" ("Substring")) -> (w357:string)
        n82 = case shown="\"d\", Default" w345 {
          tunnel: [w367 w368] -> w343
          frame "s" {
            w367 = u16 0 items=["Single", "Double"] ("sweep mode")
          }
          frame "d", Default {
            w368 = u16 1 items=["Single", "Double"] ("sweep mode")
          }
        }
        n83 = Fract/Exp String To Number(string=w344) -> (number=w339:dbl[])  [unwired: 3 in, 1 out]
        n84 = String To Path(string=w357) -> (path=w353:path)
        n85 = Index Array(array=w339, index #1=0 ("Index")) -> (element #1=w316:dbl, element #2=w315:dbl, element #3=w312:dbl, element #4=w311:dbl, element #5=w310:dbl, element #6=w314:dbl)  [unwired: 5 in]
        n86 = Bundle By Name(cluster=w313, "Pulse period"=w311, "Base voltage"=w312, "Pulse width"=w310) -> (w309:T5)
        n87 = Unbundle By Name(w309) -> ("Pulse period"=w317:dbl)
        n88 = Bundle By Name(cluster=w341, "Gate Start"=w315, "Gate Stop"=w316, "Gate Step (linear only)"=0, "Gate Compliance"=w351, "Range mode"=w331, "Range"=w330) -> (w332:T3)
        n89 = call <vilib>:"compatOverwrite.vi"("overwrite (F)"=TRUE) -> ("overwrite?"=w302:T7)
        n90 = Bundle By Name(cluster=w340, "Drain Start"=w314, "Drain Stop"=w307, "Drain Step"=w307, "Drain Compliance"=w352, "Range mode"=w329, "Range"=w328) -> (w333:T4)
        n91 = call "4155C PulsedStressV.vi"("VISA resource name in"=w335, "sweep mode"=w343, "Panel Controls"=w326, "Gate"=w332, "Drain"=w333, "Timings"=w309, "error in (no error)"=w336, "SMU4"=w325) -> ("VISA Resource Name out"=w349:refnum<visa-resource-name>, "ID"=w305:dbl[], "IG"=w303:dbl[], "Outparams"=w327:T8, "error out"=w350:errorcluster)  [unwired: 3 in]
        n92 = Unbundle By Name(w327) -> ("Number of points"=w304:i32)  [unwired: 2 out]
        n93 = for {
          N: w304 -> [_]
          tunnel: [w364] -> w306 mode=indexing
          tunnel: w317 -> [w366]
          i -> [w365]
          n94 = Multiply(x=w366, y=w365) -> (x*y=w364:dbl)
        }
        n95 = Insert Into Array(array=dbl[][] [] ("Input Array"), new element=w306) -> (w318:dbl[][])  [unwired: 2 in]
        n96 = Insert Into Array(array=w318, new element=w305) -> (w323:dbl[][])  [unwired: 2 in]
        n97 = Insert Into Array(array=w323, new element=w303) -> (w322:dbl[][])  [unwired: 2 in]
        n98 = Transpose 2D Array(2D array=w322) -> (transposed array=w321:dbl[][])
        n99 = Open/Create/Replace File(file path (use dialog)=w353, error in=w350, operation (0:open)=w302) -> (refnum out=w361:refnum<file>, error out=w362:errorcluster)  [unwired: 3 in, 1 out]
        n100 = call "4155C Write array to file.vi"("Byte Stream File Refnum"=w361, "Header"=string[] ["Time /s", "Id /A", "Ig /A"], "Data Array"=w321, "error in (no error)"=w362) -> ("dup refnum"=w359:refnum<file>, "error out"=w360:errorcluster)  [unwired: 1 in]
        n101 = Close File(refnum=w359, error in=w360) -> (error out=w348:errorcluster)  [unwired: 1 out]
      }
      frame "transfer-fpp" {
        n102 = Number To Decimal String(number=w373) -> (decimal integer string=w427:string)  [unwired: 1 in]
        n103 = Bundle By Name(cluster=w403, "Emergency Stop"=w431) -> (w439:T6)
        n104 = Delete From Array(array=w418, index=0 ("Index")) -> (deleted portion=w416:string, array with subset deleted=w415:string[])  [unwired: 1 in]
        n105 = Concatenate Strings(w426, "-transferfpp-" ("Substring"), w427, w371, ".txt" ("Substring")) -> (w429:string)
        n106 = VISA Write(VISA resource name=w395, write buffer=":PAGE:CHAN:MODE SWE;" ("write buffer (\"\")"), error in (no error)=w394) -> (VISA resource name out=w392:refnum<visa-resource-name>, error out=w393:errorcluster)  [unwired: 1 out]
        n107 = case shown="\"d\", Default" w416 {
          tunnel: [w440 w441] -> w414
          frame "s" {
            w440 = u16 0 items=["Single", "Double"] ("sweep mode")
          }
          frame "d", Default {
            w441 = u16 1 items=["Single", "Double"] ("sweep mode")
          }
        }
        n108 = Fract/Exp String To Number(string=w415) -> (number=w399:dbl[])  [unwired: 3 in, 1 out]
        n109 = String To Path(string=w429) -> (path=w425:path)
        n110 = Index Array(array=w399, index #1=0 ("Index")) -> (element #1=w413:dbl, element #2=w412:dbl, element #3=w411:dbl)  [unwired: 2 in]
        n111 = Delete From Array(array=w399, length=3 ("Length"), index=0 ("Index")) -> (array with subset deleted=w397:dbl[])  [unwired: 1 out]
        n112 = Bundle By Name(cluster=w405, "Gate Start"=w413, "Gate Stop"=w412, "Gate Step (linear only)"=w411, "Gate Compliance"=w423, "Range mode"=w388, "Range"=w387) -> (w389:T3)
        n113 = Index Array(array=w397, index #1=0 ("Index")) -> (element #1=w408:dbl, element #2=w407:dbl, element #3=w406:dbl)  [unwired: 2 in]
        n114 = call <vilib>:"compatOverwrite.vi"("overwrite (F)"=TRUE) -> ("overwrite?"=w376:T7)
        n115 = Bundle By Name(cluster=w404, "Drain Start"=w408, "Drain Stop"=w407, "Drain Step"=w406, "Drain Compliance"=w424, "Range mode"=w386, "Range"=w385) -> (w390:T4)
        n116 = call "4155C Transfer-FPP.vi"("VISA resource name in"=w392, "Gate"=w389, "Drain"=w390, "Timings"=w422, "error in (no error)"=w393, "sweep mode"=w414, "Panel Controls"=w439) -> ("VG"=w430:dbl[], "Outparams"=w384:T8, "VISA Resource Name out"=w420:refnum<visa-resource-name>, "Vprobe2"=w380:dbl[], "ID"=w379:dbl[], "IG"=w378:dbl[], "Vprobe1"=w377:dbl[], "error out"=w421:errorcluster)  [unwired: 13 in]
        n117 = Unbundle By Name(w384) -> ("V2 Step"=w383:dbl, "V2 Start"=w382:dbl, "Number of points"=w381:i32)
        n118 = Open/Create/Replace File(file path (use dialog)=w425, error in=w421, operation (0:open)=w376) -> (refnum out=w436:refnum<file>, error out=w437:errorcluster)  [unwired: 3 in, 1 out]
        n119 = call "4155C Make Big 2d array FPP.vi"("1D Var1"=w430, "1d ID"=w379, "1d Vp2"=w380, "1d IG"=w378, "1d Vp1"=w377, "VAR2 START"=w382, "Number of VAR2 steps"=w381, "VAR2 STEP"=w383, "VAR1 Name"="Vg", "Decimal places in header"=i8 1, "VAR2 Name"="Vd") -> ("Header array"=w432:string[], "Data array"=w433:dbl[][])  [unwired: 15 in]
        n120 = call "4155C Write array to file.vi"("Byte Stream File Refnum"=w436, "Header"=w432, "Data Array"=w433, "error in (no error)"=w437) -> ("dup refnum"=w434:refnum<file>, "error out"=w435:errorcluster)  [unwired: 1 in]
        n121 = Close File(refnum=w434, error in=w435) -> (error out=w419:errorcluster)  [unwired: 1 out]
      }
      frame "output" {
        n122 = Number To Decimal String(number=w454) -> (decimal integer string=w503:string)  [unwired: 1 in]
        n123 = Bundle By Name(cluster=w480, "Emergency Stop"=w506) -> (w516:T6)
        n124 = Delete From Array(array=w495, index=0 ("Index")) -> (deleted portion=w493:string, array with subset deleted=w492:string[])  [unwired: 1 in]
        n125 = Concatenate Strings(w502, "-output-" ("Substring"), w503, w453, ".txt" ("Substring")) -> (w505:string)
        n126 = VISA Write(VISA resource name=w471, write buffer=":PAGE:CHAN:MODE SWE;" ("write buffer (\"\")"), error in (no error)=w468) -> (VISA resource name out=w470:refnum<visa-resource-name>, error out=w469:errorcluster)  [unwired: 1 out]
        n127 = case shown="\"d\", Default" w493 {
          tunnel: [w517 w518] -> w491
          frame "s" {
            w517 = u16 0 items=["Single", "Double"] ("sweep mode")
          }
          frame "d", Default {
            w518 = u16 1 items=["Single", "Double"] ("sweep mode")
          }
        }
        n128 = Fract/Exp String To Number(string=w492) -> (number=w474:dbl[])  [unwired: 3 in, 1 out]
        n129 = String To Path(string=w505) -> (path=w501:path)
        n130 = Index Array(array=w474, index #1=0 ("Index")) -> (element #1=w490:dbl, element #2=w489:dbl, element #3=w488:dbl)  [unwired: 2 in]
        n131 = Delete From Array(array=w474, length=3 ("Length"), index=0 ("Index")) -> (array with subset deleted=w473:dbl[])  [unwired: 1 out]
        n132 = control-ref of="I vs Vd"() -> (w444:refnum<vi>)
        n133 = Bundle By Name(cluster=w482, "Gate Start"=w490, "Gate Stop"=w489, "Gate Step (linear only)"=w488, "Gate Compliance"=w499, "Range mode"=w466, "Range"=w465) -> (w515:T3)
        n134 = Index Array(array=w473, index #1=0 ("Index")) -> (element #1=w485:dbl, element #2=w484:dbl, element #3=w483:dbl)  [unwired: 2 in]
        n135 = call <vilib>:"compatOverwrite.vi"("overwrite (F)"=TRUE) -> ("overwrite?"=w458:T7)
        n136 = Bundle By Name(cluster=w481, "Drain Start"=w485, "Drain Stop"=w484, "Drain Step"=w483, "Drain Compliance"=w500, "Range mode"=w464, "Range"=w467) -> (w514:T4)
        n137 = call "4155C Output.vi"("VISA resource name in"=w470, "Gate"=w515, "Drain"=w514, "Timings"=w498, "error in (no error)"=w469, "SMU4"=w460, "sweep mode"=w491, "Panel controls"=w516) -> ("VD"=w451:dbl[], "Outparams"=w462:T8, "VISA Resource Name out"=w497:refnum<visa-resource-name>, "IS"=w450:dbl[], "ID"=w449:dbl[], "IG"=w448:dbl[], "error out"=w446:errorcluster, "SMU4"=w459:dbl[])  [unwired: 12 in]
        n138 = Unbundle By Name(w462) -> ("V2 Step"=w463:dbl, "V2 Start"=w461:dbl, "Number of points"=w443:i32)
        n139 = call "4155C Split array.vi"("Number of VAR2 steps"=w443, "Y2 data in"=w449, "X data in"=w451, "Y1 data in"=w450, "Y3 data in"=w448, "error in (no error)"=w446) -> ("Array of clusters"=w447:cluster{"Y data in":dbl[], "X data in":dbl[]}[], "error out"=w445:errorcluster)  [unwired: 1 in]
        n140 = local write "I vs Vd"(w447) -> ()
        n141 = call "4155C Config Chart Colours.vi"("Numeric"=w443, "XY Graph 2"=w444) -> ()  [unwired: 6 in]
        n142 = Open/Create/Replace File(file path (use dialog)=w501, error in=w445, operation (0:open)=w458) -> (refnum out=w511:refnum<file>, error out=w512:errorcluster)  [unwired: 3 in, 1 out]
        n143 = call "4155C Make Big 2d array.vi"("1D Var1"=w451, "1d IS"=w450, "1d ID"=w449, "1d IG"=w448, "1d SMU4"=w459, "SMU4"=w460, "VAR2 START"=w461, "Number of VAR2 steps"=w443, "VAR2 STEP"=w463, "VAR1 Name"="Vd", "Decimal places in header"=i8 1, "VAR2 Name"="Vg") -> ("Header array"=w507:string[], "Data array"=w508:dbl[][])  [unwired: 14 in]
        n144 = call "4155C Write array to file.vi"("Byte Stream File Refnum"=w511, "Header"=w507, "Data Array"=w508, "error in (no error)"=w512) -> ("dup refnum"=w509:refnum<file>, "error out"=w510:errorcluster)  [unwired: 1 in]
        n145 = Close File(refnum=w509, error in=w510) -> (error out=w496:errorcluster)  [unwired: 1 out]
      }
      frame "output-fpp" {
        n146 = Number To Decimal String(number=w522) -> (decimal integer string=w576:string)  [unwired: 1 in]
        n147 = Bundle By Name(cluster=w552, "Emergency Stop"=w579) -> (w589:T6)
        n148 = Delete From Array(array=w567, index=0 ("Index")) -> (deleted portion=w565:string, array with subset deleted=w564:string[])  [unwired: 1 in]
        n149 = VISA Write(VISA resource name=w543, write buffer=":PAGE:CHAN:MODE SWE;" ("write buffer (\"\")"), error in (no error)=w540) -> (VISA resource name out=w542:refnum<visa-resource-name>, error out=w541:errorcluster)  [unwired: 1 out]
        n150 = Concatenate Strings(w575, "-outputfpp-" ("Substring"), w576, w521, ".txt" ("Substring")) -> (w578:string)
        n151 = case shown="\"d\", Default" w565 {
          tunnel: [w590 w591] -> w563
          frame "s" {
            w590 = u16 0 items=["Single", "Double"] ("sweep mode")
          }
          frame "d", Default {
            w591 = u16 1 items=["Single", "Double"] ("sweep mode")
          }
        }
        n152 = Fract/Exp String To Number(string=w564) -> (number=w546:dbl[])  [unwired: 3 in, 1 out]
        n153 = String To Path(string=w578) -> (path=w574:path)
        n154 = Index Array(array=w546, index #1=0 ("Index")) -> (element #1=w562:dbl, element #2=w561:dbl, element #3=w560:dbl)  [unwired: 2 in]
        n155 = Delete From Array(array=w546, length=3 ("Length"), index=0 ("Index")) -> (array with subset deleted=w545:dbl[])  [unwired: 1 out]
        n156 = Bundle By Name(cluster=w554, "Gate Start"=w562, "Gate Stop"=w561, "Gate Step (linear only)"=w560, "Gate Compliance"=w572, "Range mode"=w538, "Range"=w537) -> (w588:T3)
        n157 = Index Array(array=w545, index #1=0 ("Index")) -> (element #1=w557:dbl, element #2=w556:dbl, element #3=w555:dbl)  [unwired: 2 in]
        n158 = call <vilib>:"compatOverwrite.vi"("overwrite (F)"=TRUE) -> ("overwrite?"=w526:T7)
        n159 = Bundle By Name(cluster=w553, "Drain Start"=w557, "Drain Stop"=w556, "Drain Step"=w555, "Drain Compliance"=w573, "Range mode"=w536, "Range"=w539) -> (w587:T4)
        n160 = call "4155C Output-FPP.vi"("VISA resource name in"=w542, "Gate"=w588, "Drain"=w587, "Timings"=w571, "error in (no error)"=w541, "sweep mode"=w563, "Panel controls"=w589) -> ("VD"=w531:dbl[], "Outparams"=w534:T8, "VISA Resource Name out"=w569:refnum<visa-resource-name>, "Vprobe2"=w530:dbl[], "ID"=w529:dbl[], "IG"=w528:dbl[], "Vprobe1"=w527:dbl[], "error out"=w570:errorcluster)  [unwired: 13 in]
        n161 = Unbundle By Name(w534) -> ("V2 Step"=w535:dbl, "V2 Start"=w533:dbl, "Number of points"=w532:i32)
        n162 = Open/Create/Replace File(file path (use dialog)=w574, error in=w570, operation (0:open)=w526) -> (refnum out=w584:refnum<file>, error out=w585:errorcluster)  [unwired: 3 in, 1 out]
        n163 = call "4155C Make Big 2d array FPP.vi"("1D Var1"=w531, "1d ID"=w529, "1d Vp2"=w530, "1d IG"=w528, "1d Vp1"=w527, "VAR2 START"=w533, "Number of VAR2 steps"=w532, "VAR2 STEP"=w535, "VAR1 Name"="Vd", "Decimal places in header"=i8 1, "VAR2 Name"="Vg") -> ("Header array"=w580:string[], "Data array"=w581:dbl[][])  [unwired: 15 in]
        n164 = call "4155C Write array to file.vi"("Byte Stream File Refnum"=w584, "Header"=w580, "Data Array"=w581, "error in (no error)"=w585) -> ("dup refnum"=w582:refnum<file>, "error out"=w583:errorcluster)  [unwired: 1 in]
        n165 = Close File(refnum=w582, error in=w583) -> (error out=w568:errorcluster)  [unwired: 1 out]
      }
      frame "itime" {
        n166 = Delete From Array(array=w607, index=0 ("Index")) -> (deleted portion=w608:string)  [unwired: 1 in, 1 out]
        n167 = case shown="\"l\"" w608 {
          tunnel: w606 -> [w612 w614 w617]
          tunnel: [w611 w613 w616] -> w599
          frame "s" {
            w610 = u32 0 items=["short  ", "medium  ", "long  "] ("integration time 2")
            n168 = Bundle By Name(cluster=w612, "integration time"=w610) -> (w611:T5)
          }
          frame "m", Default {
            w615 = u32 1 items=["short  ", "medium  ", "long  "] ("integration time 2")
            n169 = Bundle By Name(cluster=w614, "integration time"=w615) -> (w613:T5)
          }
          frame "l" {
            w618 = u32 2 items=["short  ", "medium  ", "long  "] ("integration time 2")
            n170 = Bundle By Name(cluster=w617, "integration time"=w618) -> (w616:T5)
          }
        }
      }
      frame "pulsed" {
        n171 = Delete From Array(array=w635, index=0 ("Index")) -> (deleted portion=w636:string, array with subset deleted=w623:string[])  [unwired: 1 in]
        n172 = case shown="\"on\", Default" w636 {
          tunnel: w634 -> [w646 w649]
          tunnel: [w645 w648] -> w627
          tunnel: w623 -> [w643 _]
          frame "on", Default {
            w644 = u16 1 items=["Continuous", "Pulsed"] ("sweep method")
            n173 = Fract/Exp String To Number(string=w643) -> (number=w641:dbl[])  [unwired: 3 in, 1 out]
            n174 = Index Array(array=w641, index #1=0 ("Index")) -> (element #1=w640:dbl, element #2=w639:dbl, element #3=w638:dbl)  [unwired: 2 in]
            n175 = Bundle By Name(cluster=w646, "sweep method"=w644, "Pulse period"=w640, "Base voltage"=w639, "Pulse width"=w638) -> (w645:T5)
          }
          frame "off" {
            w647 = u16 0 items=["Continuous", "Pulsed"] ("sweep method")
            n176 = Bundle By Name(cluster=w649, "sweep method"=w647) -> (w648:T5)
          }
        }
      }
      frame "gaterangemode" {
        n177 = Delete From Array(array=w664, index=0 ("Index")) -> (deleted portion=w665:string)  [unwired: 1 in, 1 out]
        n178 = case shown="\"f\"" w665 {
          tunnel: [w667 w668 w669] -> w654
          frame "a", Default {
            w667 = u16 0 items=["Auto", "Limited", "Fixed"] ("Gate Range\nmode 2")
          }
          frame "f" {
            w668 = u16 2 items=["Auto", "Limited", "Fixed"] ("Gate Range\nmode 2")
          }
          frame "l" {
            w669 = u16 1 items=["Auto", "Limited", "Fixed"] ("Gate Range\nmode 2")
          }
        }
      }
      frame "gaterange" {
        (unwired) u8 11 items=["10fA  ", "100fA  ", "1nA  ", "10nA", "100nA", "1uA", "10uA", "100uA", "1mA", "10mA", "100mA", "1A"] ("Gate Range 2")
        n179 = Delete From Array(array=w691, index=0 ("Index")) -> (deleted portion=w681:string)  [unwired: 1 in, 1 out]
        n180 = Scan Value(string=w681, format string="") -> (value=w679:dbl)  [unwired: 1 in, 1 out]
        n181 = Logarithm Base 10(1:w679) -> (0:w678:dbl)
        n182 = Round To Nearest(number=w678) -> (nearest integer value=w677:dbl)
        n183 = Add(x=w677, y=11.0) -> (x+y=w675:dbl)
        n184 = To Unsigned Byte Integer(number=w675) -> (unsigned 8bit integer=w674:u8)
      }
      frame "drainrange" {
        (unwired) u8 11 items=["10fA  ", "100fA  ", "1nA  ", "10nA", "100nA", "1uA", "10uA", "100uA", "1mA", "10mA", "100mA", "1A"] ("Gate Range 2")
        n185 = Delete From Array(array=w714, index=0 ("Index")) -> (deleted portion=w705:string)  [unwired: 1 in, 1 out]
        n186 = Scan Value(string=w705, format string="") -> (value=w703:dbl)  [unwired: 1 in, 1 out]
        n187 = Logarithm Base 10(1:w703) -> (0:w702:dbl)
        n188 = Round To Nearest(number=w702) -> (nearest integer value=w701:dbl)
        n189 = Add(x=w701, y=11.0) -> (x+y=w699:dbl)
        n190 = To Unsigned Byte Integer(number=w699) -> (unsigned 8bit integer=w698:u8)
      }
      frame "drainrangemode" {
        n191 = Delete From Array(array=w730, index=0 ("Index")) -> (deleted portion=w731:string)  [unwired: 1 in, 1 out]
        n192 = case shown="\"f\"" w731 {
          tunnel: [w733 w734 w735] -> w720
          frame "a", Default {
            w733 = u16 0 items=["Auto", "Limited", "Fixed"] ("Gate Range\nmode 2")
          }
          frame "f" {
            w734 = u16 2 items=["Auto", "Limited", "Fixed"] ("Gate Range\nmode 2")
          }
          frame "l" {
            w735 = u16 1 items=["Auto", "Limited", "Fixed"] ("Gate Range\nmode 2")
          }
        }
      }
      frame "Error", Default {
      }
      frame "logfile" {
        n193 = Number To Decimal String(number=w754) -> (decimal integer string=w789:string)  [unwired: 1 in]
        n194 = Concatenate Strings(w788, "logfile" ("Substring"), w789, w752, ".txt" ("Substring")) -> (w786:string)
        n195 = String To Path(string=w786) -> (path=w759:path)
        n196 = Unbundle(w785) -> ("integration time"=w784:u32, "Short/Long integration time"=w783:dbl, "hold time (sec)"=w782:dbl, "delay time (sec)"=w781:dbl, "Step Time (0 disables)"=w780:dbl, "sweep method"=w779:u16, "Pulse period"=w778:dbl, "Base voltage"=w777:dbl, "Pulse width"=w776:dbl)
        n197 = Build Array(w784, w783, w782, w781, w780, w779, w778, w777, w776, w770, w771, w772, w773, w774, w775) -> (w763:dbl[])
        n198 = Insert Into Array(array=dbl[][] [] ("Input Array"), new element=w763) -> (w762:dbl[][])  [unwired: 2 in]
        n199 = call <vilib>:"compatOverwrite.vi"("overwrite (F)"=TRUE) -> ("overwrite?"=w757:T7)
        n200 = Open/Create/Replace File(file path (use dialog)=w759, error in=w761, operation (0:open)=w757) -> (refnum out=w767:refnum<file>, error out=w766:errorcluster)  [unwired: 3 in, 1 out]
        n201 = call "4155C Write array to file.vi"("Byte Stream File Refnum"=w767, "Header"=string[] ["Int Time", "Short/Long Itime", "Hold time", "Delay time", "Step time", "Sweep method", "Pulse period", "Base Voltage", "Pulse width", "Drain compliance", "Gate compliance", "Gate range mode", "Gate range", "S/D range mode", "S/D range"], "Data Array"=w762, "error in (no error)"=w766) -> ("dup refnum"=w769:refnum<file>, "error out"=w768:errorcluster)  [unwired: 1 in]
        n202 = Close File(refnum=w769, error in=w768) -> (error out=w760:errorcluster)  [unwired: 1 out]
      }
      frame "sample" {
        n203 = Number To Decimal String(number=w795) -> (decimal integer string=w843:string)  [unwired: 1 in]
        n204 = Fract/Exp String To Number(string=w840) -> (number=w801:dbl[])  [unwired: 3 in, 1 out]
        n205 = Concatenate Strings(w818, "-sample-" ("Substring"), w843, w793, ".txt" ("Substring")) -> (w841:string)
        n206 = String To Path(string=w841) -> (path=w822:path)
        n207 = Index Array(array=w801, index=0 ("Index")) -> (element=w838:dbl)
        n208 = Index Array(array=w801, index=2 ("Index")) -> (element=w834:dbl)
        n209 = Index Array(array=w801, index=3 ("Index")) -> (element=w803:dbl)
        n210 = Index Array(array=w801, index=4 ("Index")) -> (element=w800:dbl)
        n211 = call "4155C Config Sampling Measurements.vi"("Sampling interval"=w800, "Sample time"=w803, "Display on/off"=TRUE, "Timings"=w809, "Num Points"=w834, "error in (no error)"=w845, "Drain Compliance"=w844, "Gate Compliance"=w819, "VISA session"=w846) -> ("error out"=w847:errorcluster, "dup VISA resource name"=w848:refnum<visa-resource-name>)  [unwired: 1 in]
        n212 = Index Array(array=w801, index=1 ("Index")) -> (element=w835:dbl)
        n213 = call "4155C Take Sample.vi"("Emergency Stop"=w815, "error in (no error)"=w847, "Vd"=w835, "Vg"=w838, "VISA resource name in"=w848) -> ("error out"=w813:errorcluster, "Id"=w850:dbl[], "Ig"=w824:dbl[], "VISA Resource Name out"=w811:refnum<visa-resource-name>, "Is"=w849:dbl[], "Time"=w828:dbl[])  [unwired: 1 in]
        n214 = Insert Into Array(array=dbl[][] [] ("Input Array"), new element=w828) -> (w827:dbl[][])  [unwired: 2 in]
        n215 = Insert Into Array(array=w827, new element=w824) -> (w826:dbl[][])  [unwired: 2 in]
        n216 = Insert Into Array(array=w826, new element=w850) -> (w825:dbl[][])  [unwired: 2 in]
        n217 = VISA Write(VISA resource name=w811, write buffer=":DISP ON" ("write buffer (\"\")"), error in (no error)=w813) -> (VISA resource name out=w810:refnum<visa-resource-name>, error out=w812:errorcluster)  [unwired: 1 out]
        n218 = Insert Into Array(array=w825, new element=w849) -> (w817:dbl[][])  [unwired: 2 in]
        n219 = Transpose 2D Array(2D array=w817) -> (transposed array=w816:dbl[][])
        n220 = call <vilib>:"compatOverwrite.vi"("overwrite (F)"=TRUE) -> ("overwrite?"=w798:T7)
        n221 = Open/Create/Replace File(file path (use dialog)=w822, error in=w812, operation (0:open)=w798) -> (refnum out=w831:refnum<file>, error out=w830:errorcluster)  [unwired: 3 in, 1 out]
        n222 = call "4155C Write array to file.vi"("Byte Stream File Refnum"=w831, "Header"=string[] ["Time /s", "Ig /A", "Id /A", "Is /A"], "Data Array"=w816, "error in (no error)"=w830) -> ("dup refnum"=w833:refnum<file>, "error out"=w832:errorcluster)  [unwired: 1 in]
        n223 = Close File(refnum=w833, error in=w832) -> (error out=w820:errorcluster)  [unwired: 1 out]
      }
      frame "samplei" {
        n224 = Number To Decimal String(number=w854) -> (decimal integer string=w906:string)  [unwired: 1 in]
        n225 = Fract/Exp String To Number(string=w903) -> (number=w870:dbl[])  [unwired: 3 in, 1 out]
        n226 = Concatenate Strings(w885, "-samplei-" ("Substring"), w906, w853, ".txt" ("Substring")) -> (w904:string)
        n227 = String To Path(string=w904) -> (path=w888:path)
        n228 = Index Array(array=w870, index=4 ("Index")) -> (element=w864:dbl)
        n229 = Index Array(array=w870, index=3 ("Index")) -> (element=w865:dbl)
        n230 = Index Array(array=w870, index=1 ("Index")) -> (element=w867:dbl)
        n231 = Index Array(array=w870, index=0 ("Index")) -> (element=w868:dbl)
        n232 = Index Array(array=w870, index=2 ("Index")) -> (element=w866:dbl)
        n233 = call "4155C Config SamplingI Measurements.vi"("Sample time"=w866, "Display on/off"=TRUE, "Timings"=w877, "Num Points"=w867, "error in (no error)"=w908, "Sampling interval"=w865, "VISA session"=w909) -> ("error out"=w910:errorcluster, "dup VISA resource name"=w911:refnum<visa-resource-name>)  [unwired: 3 in]
        n234 = call "4155C Take SampleI.vi"("Emergency Stop"=w882, "error in (no error)"=w910, "Idg 2"=w868, "Vdg compliance 2"=w864, "VISA resource name in"=w911) -> ("error out"=w880:errorcluster, "Idg"=w913:dbl[], "Vdg"=w890:dbl[], "VISA Resource Name out"=w878:refnum<visa-resource-name>, "Is"=w912:dbl[], "Time"=w894:dbl[])  [unwired: 1 in]
        n235 = Insert Into Array(array=dbl[][] [] ("Input Array"), new element=w894) -> (w893:dbl[][])  [unwired: 2 in]
        n236 = Insert Into Array(array=w893, new element=w890) -> (w892:dbl[][])  [unwired: 2 in]
        n237 = Insert Into Array(array=w892, new element=w913) -> (w891:dbl[][])  [unwired: 2 in]
        n238 = VISA Write(VISA resource name=w878, write buffer=":DISP ON" ("write buffer (\"\")"), error in (no error)=w880) -> (VISA resource name out=w863:refnum<visa-resource-name>, error out=w879:errorcluster)  [unwired: 1 out]
        n239 = Insert Into Array(array=w891, new element=w912) -> (w884:dbl[][])  [unwired: 2 in]
        n240 = Transpose 2D Array(2D array=w884) -> (transposed array=w883:dbl[][])
        n241 = call <vilib>:"compatOverwrite.vi"("overwrite (F)"=TRUE) -> ("overwrite?"=w858:T7)
        n242 = Open/Create/Replace File(file path (use dialog)=w888, error in=w879, operation (0:open)=w858) -> (refnum out=w897:refnum<file>, error out=w896:errorcluster)  [unwired: 3 in, 1 out]
        n243 = call "4155C Write array to file.vi"("Byte Stream File Refnum"=w897, "Header"=string[] ["Time /s", "Vdg /V", "Idg /A", "Is /A"], "Data Array"=w883, "error in (no error)"=w896) -> ("dup refnum"=w899:refnum<file>, "error out"=w898:errorcluster)  [unwired: 1 in]
        n244 = Close File(refnum=w899, error in=w898) -> (error out=w861:errorcluster)  [unwired: 1 out]
        n245 = VISA Write(VISA resource name=w863, write buffer=";:PAGE:SCON:STAN OFF;:PAGE:CHAN:VSU2:DIS;" ("write buffer (\"\")"), error in (no error)=w861) -> (VISA resource name out=w859:refnum<visa-resource-name>, error out=w860:errorcluster)  [unwired: 1 out]
      }
      frame "#" {
        n246 = VISA Write(VISA resource name=w922, write buffer=":DISP ON" ("write buffer (\"\")"), error in (no error)=w921) -> (VISA resource name out=w920:refnum<visa-resource-name>, error out=w919:errorcluster)  [unwired: 1 out]
      }
      frame "stressV" {
        n247 = Number To Decimal String(number=w934) -> (decimal integer string=w975:string)  [unwired: 1 in]
        n248 = Fract/Exp String To Number(string=w972) -> (number=w945:dbl[])  [unwired: 3 in, 1 out]
        n249 = Concatenate Strings(w959, "-stressV-" ("Substring"), w975, w933, ".txt" ("Substring")) -> (w973:string)
        n250 = String To Path(string=w973) -> (path=w963:path)
        n251 = Index Array(array=w945, index=3 ("Index")) -> (element=w942:dbl)
        n252 = Index Array(array=w945, index=1 ("Index")) -> (element=w940:dbl)
        n253 = Index Array(array=w945, index=0 ("Index")) -> (element=w939:dbl)
        n254 = Index Array(array=w945, index=4 ("Index")) -> (element=w944:dbl)
        n255 = Index Array(array=w945, index=2 ("Index")) -> (element=w941:dbl)
        n256 = call "4155C Config V Stress.vi"("VISA session"=w978, "ID compliance"=w942, "VD"=w940, "VG"=w939, "IG compliance"=w941, "error in (no error)"=w977, "Display on/off"=TRUE) -> ("dup VISA resource name"=w980:refnum<visa-resource-name>, "error out"=w979:errorcluster)
        n257 = call "4155C Apply Stress.vi"("error in (no error)"=w979, "Duration"=w944, "Emergency Stop"=w958, "VISA resource name in"=w980) -> ("error out"=w956:errorcluster, "VISA Resource Name out"=w954:refnum<visa-resource-name>)
        n258 = VISA Write(VISA resource name=w954, write buffer=":DISP ON" ("write buffer (\"\")"), error in (no error)=w956) -> (VISA resource name out=w953:refnum<visa-resource-name>, error out=w955:errorcluster)  [unwired: 1 out]
        n259 = call <vilib>:"compatOverwrite.vi"("overwrite (F)"=TRUE) -> ("overwrite?"=w938:T7)
        n260 = Open/Create/Replace File(file path (use dialog)=w963, error in=w955, operation (0:open)=w938) -> (refnum out=w966:refnum<file>, error out=w965:errorcluster)  [unwired: 3 in, 1 out]
        n261 = call "4155C Write array to file.vi"("Byte Stream File Refnum"=w966, "Header"=string[] ["V stress completed successfully", ""], "error in (no error)"=w965) -> ("dup refnum"=w968:refnum<file>, "error out"=w967:errorcluster)  [unwired: 2 in]
        n262 = Close File(refnum=w968, error in=w967) -> (error out=w961:errorcluster)  [unwired: 1 out]
      }
      frame "stressI" {
        n263 = Number To Decimal String(number=w984) -> (decimal integer string=w1021:string)  [unwired: 1 in]
        n264 = Fract/Exp String To Number(string=w1018) -> (number=w993:dbl[])  [unwired: 3 in, 1 out]
        n265 = Concatenate Strings(w1005, "-stressI-" ("Substring"), w1021, w983, ".txt" ("Substring")) -> (w1019:string)
        n266 = String To Path(string=w1019) -> (path=w1009:path)
        n267 = Index Array(array=w993, index=1 ("Index")) -> (element=w989:dbl)
        n268 = Index Array(array=w993, index=0 ("Index")) -> (element=w990:dbl)
        n269 = call "4155C Config I Stress.vi"("VISA session"=w1024, "IDG"=w990, "VDG compliance"=w989, "error in (no error)"=w1023, "Display on/off"=TRUE) -> ("dup VISA resource name"=w1026:refnum<visa-resource-name>, "error out"=w1025:errorcluster)
        n270 = Index Array(array=w993, index=2 ("Index")) -> (element=w991:dbl)
        n271 = call "4155C Apply Stress.vi"("error in (no error)"=w1025, "Duration"=w991, "Emergency Stop"=w1004, "VISA resource name in"=w1026) -> ("error out"=w1002:errorcluster, "VISA Resource Name out"=w1000:refnum<visa-resource-name>)
        n272 = VISA Write(VISA resource name=w1000, write buffer=":DISP ON" ("write buffer (\"\")"), error in (no error)=w1002) -> (VISA resource name out=w999:refnum<visa-resource-name>, error out=w1001:errorcluster)  [unwired: 1 out]
        n273 = call <vilib>:"compatOverwrite.vi"("overwrite (F)"=TRUE) -> ("overwrite?"=w988:T7)
        n274 = Open/Create/Replace File(file path (use dialog)=w1009, error in=w1001, operation (0:open)=w988) -> (refnum out=w1012:refnum<file>, error out=w1011:errorcluster)  [unwired: 3 in, 1 out]
        n275 = call "4155C Write array to file.vi"("Byte Stream File Refnum"=w1012, "Header"=string[] ["I stress completed successfully", ""], "error in (no error)"=w1011) -> ("dup refnum"=w1014:refnum<file>, "error out"=w1013:errorcluster)  [unwired: 2 in]
        n276 = Close File(refnum=w1014, error in=w1013) -> (error out=w1007:errorcluster)  [unwired: 1 out]
      }
      frame "vsu2pulse" {
        n277 = Number To Decimal String(number=w1030) -> (decimal integer string=w1065:string)  [unwired: 1 in]
        n278 = Fract/Exp String To Number(string=w1062) -> (number=w1038:dbl[])  [unwired: 3 in, 1 out]
        n279 = Concatenate Strings(w1050, "-vsu2-" ("Substring"), w1065, w1029, ".txt" ("Substring")) -> (w1063:string)
        n280 = String To Path(string=w1063) -> (path=w1054:path)
        n281 = Index Array(array=w1038, index=1 ("Index")) -> (element=w1037:dbl)
        n282 = Index Array(array=w1038, index=0 ("Index")) -> (element=w1035:dbl)
        n283 = call "4155C Config VSU2 Stress.vi"("error in (no error)"=w1067, "VSU2"=w1035, "Display on/off"=TRUE, "VISA session"=w1068) -> ("error out"=w1069:errorcluster, "dup VISA resource name"=w1070:refnum<visa-resource-name>)
        n284 = call "4155C Apply Stress.vi"("error in (no error)"=w1069, "Duration"=w1037, "Emergency Stop"=w1049, "VISA resource name in"=w1070) -> ("error out"=w1047:errorcluster, "VISA Resource Name out"=w1045:refnum<visa-resource-name>)
        n285 = VISA Write(VISA resource name=w1045, write buffer=":DISP ON" ("write buffer (\"\")"), error in (no error)=w1047) -> (VISA resource name out=w1044:refnum<visa-resource-name>, error out=w1046:errorcluster)  [unwired: 1 out]
        n286 = call <vilib>:"compatOverwrite.vi"("overwrite (F)"=TRUE) -> ("overwrite?"=w1034:T7)
        n287 = Open/Create/Replace File(file path (use dialog)=w1054, error in=w1046, operation (0:open)=w1034) -> (refnum out=w1057:refnum<file>, error out=w1056:errorcluster)  [unwired: 3 in, 1 out]
        n288 = call "4155C Write array to file.vi"("Byte Stream File Refnum"=w1057, "Header"=string[] ["VSU2 pulse completed successfully", ""], "error in (no error)"=w1056) -> ("dup refnum"=w1059:refnum<file>, "error out"=w1058:errorcluster)  [unwired: 2 in]
        n289 = Close File(refnum=w1059, error in=w1058) -> (error out=w1052:errorcluster)  [unwired: 1 out]
      }
      frame "sample-fpp" {
        w1085 = string[] ["Time /s", "Id VgVd /A", "Ig VgVd /A", "Vp1 VgVd /V", "Vp2 VgVd /V"] ("Header")
        w1089 = "%d" ("format string")
        n290 = Number To Decimal String(number=w1074) -> (decimal integer string=w1137:string)  [unwired: 1 in]
        n291 = Fract/Exp String To Number(string=w1134) -> (number=w1122:dbl[])  [unwired: 3 in, 1 out]
        n292 = Concatenate Strings(w1128, "-samplefpp-" ("Substring"), w1137, w1073, ".txt" ("Substring")) -> (w1135:string)
        n293 = String To Path(string=w1135) -> (path=w1097:path)
        n294 = Index Array(array=w1122, index=0 ("Index")) -> (element=w1083:dbl)
        n295 = Index Array(array=w1122, index=1 ("Index")) -> (element=w1082:dbl)
        n296 = Index Array(array=w1122, index=2 ("Index")) -> (element=w1130:dbl)
        n297 = Index Array(array=w1122, index=3 ("Index")) -> (element=w1120:dbl)
        n298 = call "4155C Config Sampling Measurements FPP.vi"("VISA session"=w1140, "Num Points"=w1130, "Vg"=w1083, "Display on/off"=TRUE, "Gate Compliance"=w1129, "Drain Compliance"=w1138, "Standby"="Standby", "error in (no error)"=w1139, "Timings"=w1127, "Vd"=w1082, "Sample time"=w1120) -> ("dup VISA resource name"=w1099:refnum<visa-resource-name>, "error out"=w1098:errorcluster)  [unwired: 3 in]
        n299 = Number To Decimal String(number=w1083) -> (decimal integer string=w1109:string)  [unwired: 1 in]
        n300 = call "4155C Take Sample FPP.vi"("VISA resource name in"=w1099, "error in (no error)"=w1098, "Emergency Stop"=w1100) -> ("Time"=w1104:dbl[], "Vp1"=w1114:dbl[], "VISA Resource Name out"=w1080:refnum<visa-resource-name>, "Ig"=w1102:dbl[], "Id"=w1103:dbl[], "Vp2"=w1112:dbl[], "error out"=w1101:errorcluster)  [unwired: 10 in]
        n301 = Insert Into Array(array=dbl[][] [] ("Input Array"), new element=w1104) -> (w1118:dbl[][])  [unwired: 2 in]
        n302 = Number To Decimal String(number=w1082) -> (decimal integer string=w1107:string)  [unwired: 1 in]
        n303 = Insert Into Array(array=w1118, new element=w1103) -> (w1117:dbl[][])  [unwired: 2 in]
        n304 = Concatenate Strings("(Vg = " ("Substring"), w1109, "V, Vd = " ("Substring"), w1107, "V)" ("Substring")) -> (w1105:string)
        n305 = Insert Into Array(array=w1117, new element=w1102) -> (w1116:dbl[][])  [unwired: 2 in]
        n306 = Insert Into Array(array=w1116, new element=w1114) -> (w1113:dbl[][])  [unwired: 2 in]
        n307 = Insert Into Array(array=w1113, new element=w1112) -> (w1081:dbl[][])  [unwired: 2 in]
        n308 = call <vilib>:"compatOverwrite.vi"("overwrite (F)"=TRUE) -> ("overwrite?"=w1078:T7)
        n309 = Open/Create/Replace File(file path (use dialog)=w1097, error in=w1101, operation (0:open)=w1078) -> (refnum out=w1094:refnum<file>, error out=w1095:errorcluster)  [unwired: 3 in, 1 out]
        n310 = Array To Spreadsheet String(array=w1085, 3:w1089) -> (spreadsheet string=w1091:string)  [unwired: 1 in]
        n311 = Transpose 2D Array(2D array=w1081) -> (transposed array=w1111:dbl[][])
        n312 = Search and Replace String(replace all?=TRUE ("replace all? (F)"), input string=w1091, search string="VgVd", replace string=w1105) -> (result string=w1087:string)  [unwired: 4 in, 3 out]
        n313 = Spreadsheet String To Array(format string=w1089, spreadsheet string=w1087, array type (2D Dbl)=w1085) -> (array=w1086:string[])  [unwired: 1 in]
        n314 = call "4155C Write array to file.vi"("Byte Stream File Refnum"=w1094, "Header"=w1086, "Data Array"=w1111, "error in (no error)"=w1095) -> ("dup refnum"=w1092:refnum<file>, "error out"=w1093:errorcluster)  [unwired: 1 in]
        n315 = Close File(refnum=w1092, error in=w1093) -> (error out=w1079:errorcluster)  [unwired: 1 out]
      }
      frame "resample-fpp" {
        w1157 = string[] ["Time /s", "Id VgVd /A", "Ig VgVd /A", "Vp1 VgVd /V", "Vp2 VgVd /V"] ("Header")
        w1161 = "%d" ("format string")
        n316 = Number To Decimal String(number=w1143) -> (decimal integer string=w1201:string)  [unwired: 1 in]
        n317 = Fract/Exp String To Number(string=w1198) -> (number=w1150:dbl[])  [unwired: 3 in, 1 out]
        n318 = Concatenate Strings(w1194, "-resamplefpp-" ("Substring"), w1201, w1144, ".txt" ("Substring")) -> (w1199:string)
        n319 = String To Path(string=w1199) -> (path=w1169:path)
        n320 = Index Array(array=w1150, index=0 ("Index")) -> (element=w1156:dbl)
        n321 = Index Array(array=w1150, index=1 ("Index")) -> (element=w1155:dbl)
        n322 = Number To Decimal String(number=w1156) -> (decimal integer string=w1179:string)  [unwired: 1 in]
        n323 = call "4155C Take Sample FPP.vi"("VISA resource name in"=w1152, "error in (no error)"=w1151, "Emergency Stop"=w1170) -> ("Time"=w1174:dbl[], "Vp1"=w1184:dbl[], "VISA Resource Name out"=w1154:refnum<visa-resource-name>, "Ig"=w1172:dbl[], "Id"=w1173:dbl[], "Vp2"=w1182:dbl[], "error out"=w1171:errorcluster)  [unwired: 10 in]
        n324 = Insert Into Array(array=dbl[][] [] ("Input Array"), new element=w1174) -> (w1188:dbl[][])  [unwired: 2 in]
        n325 = Number To Decimal String(number=w1155) -> (decimal integer string=w1177:string)  [unwired: 1 in]
        n326 = Insert Into Array(array=w1188, new element=w1173) -> (w1187:dbl[][])  [unwired: 2 in]
        n327 = Concatenate Strings("(Vg = " ("Substring"), w1179, "V, Vd = " ("Substring"), w1177, "V)" ("Substring")) -> (w1175:string)
        n328 = Insert Into Array(array=w1187, new element=w1172) -> (w1186:dbl[][])  [unwired: 2 in]
        n329 = Insert Into Array(array=w1186, new element=w1184) -> (w1183:dbl[][])  [unwired: 2 in]
        n330 = Insert Into Array(array=w1183, new element=w1182) -> (w1149:dbl[][])  [unwired: 2 in]
        n331 = call <vilib>:"compatOverwrite.vi"("overwrite (F)"=TRUE) -> ("overwrite?"=w1148:T7)
        n332 = Open/Create/Replace File(file path (use dialog)=w1169, error in=w1171, operation (0:open)=w1148) -> (refnum out=w1166:refnum<file>, error out=w1167:errorcluster)  [unwired: 3 in, 1 out]
        n333 = Array To Spreadsheet String(array=w1157, 3:w1161) -> (spreadsheet string=w1163:string)  [unwired: 1 in]
        n334 = Transpose 2D Array(2D array=w1149) -> (transposed array=w1181:dbl[][])
        n335 = Search and Replace String(replace all?=TRUE ("replace all? (F)"), input string=w1163, search string="VgVd", replace string=w1175) -> (result string=w1159:string)  [unwired: 4 in, 3 out]
        n336 = Spreadsheet String To Array(format string=w1161, spreadsheet string=w1159, array type (2D Dbl)=w1157) -> (array=w1158:string[])  [unwired: 1 in]
        n337 = call "4155C Write array to file.vi"("Byte Stream File Refnum"=w1166, "Header"=w1158, "Data Array"=w1181, "error in (no error)"=w1167) -> ("dup refnum"=w1164:refnum<file>, "error out"=w1165:errorcluster)  [unwired: 1 in]
        n338 = Close File(refnum=w1164, error in=w1165) -> (error out=w1153:errorcluster)  [unwired: 1 out]
      }
      frame "serial" {
        n339 = Index Array(array=w1210, index=0 ("Index")) -> (element=w1209:string)
        n340 = call "Serial write and read v0.5.vi"("Delay before read (ms)"="Delay before read (ms)", "Termination char\n(0xA = '\\n' = LF)\n(0xD = '\\r' = CR)"="Termination char\n(0xA = '\\n' = LF)\n(0xD = '\\r' = CR)", "Enable Termination\nChar (T)"="Enable Termination\nChar (T)", "parity"="parity", "stop bits"="stop bits", "string to write"=w1209, "flow control"="flow control", "byte count"="byte count", "Serial Settings:Serial End Mode for Reads"="Serial End Mode for Reads", "Timeout (ms)"="Timeout (ms)", "error in (no error)"=w1215, "VISA resource name"="VISA resource name", "baud rate"="baud rate", "data bits"="data bits") -> ("read string"=w1206:string, "error out"=w1214:errorcluster)
        n341 = Build Array (concatenate)(w1206, w1204) -> (w1205:string[])
      }
    }
    n342 = Build Array("Time /s" ("element"), "Id max /A" ("VAR2 Name"), "Id min /A" ("VAR2 Name")) -> (w85:string[])
    n343 = Build Array(w80, w79, w72) -> (w78:dbl[][])
    n344 = Concatenate Strings(w50, "-Serial port output", ".txt" ("Suffix")) -> (w54:string)
    n345 = Array To Spreadsheet String(array=w55, 3:"" ("format string")) -> (spreadsheet string=w60:string)  [unwired: 1 in]
    n346 = Transpose 2D Array(2D array=w78) -> (transposed array=w77:dbl[][])
    n347 = String To Path(string=w54) -> (path=w51:path)
    n348 = Concatenate Strings(w50, "-Ion-Ioff", ".txt" ("Suffix")) -> (w93:string)
    n349 = Array To Spreadsheet String(array=w85, 3:"" ("format string")) -> (spreadsheet string=w84:string)  [unwired: 1 in]
    n350 = Array To Spreadsheet String(array=w77, 3:"%e" ("format string")) -> (spreadsheet string=w83:string)  [unwired: 1 in]
    n351 = String To Path(string=w93) -> (path=w92:path)
    n352 = local write "Serial port output"(w60) -> ()
    n353 = Write to Text File(file (use dialog)=w51, text=w55) -> (refnum out=w56:refnum<file>, error out=w57:errorcluster)  [unwired: 2 in, 1 out]
    n354 = Build Array(w84, w83) -> (w82:string[])
    n355 = Close File(refnum=w56, error in=w57) -> ()  [unwired: 2 out]
    n356 = Write to Text File(file (use dialog)=w92, text=w82, error in=w75) -> (refnum out=w94:refnum<file>, error out=w81:errorcluster)  [unwired: 1 in, 1 out]
    n357 = Close File(refnum=w94, error in=w81) -> (error out=w74:errorcluster)  [unwired: 1 out]
  }
  "error out" <- w9
